vi "Untitled 2.vi"() -> ()   [LabVIEW 2016]
uses:
  <userlib>/LevyLab/XY Utilities/Typedefs/Interpolation Configuration--cluster.ctl
  <userlib>/LevyLab/Graph Utilities/graph_utilities.lvclass
  <userlib>/LevyLab/Graph Utilities/graph_utilities.lvclass/graph_utilities.ctl
  <userlib>/LevyLab/Graph Utilities/XY Graph/Set XY Graph Value (array).vi
  <userlib>/LevyLab/XY Utilities/subVIs/Add float (multiple).vi
  <userlib>/LevyLab/XY Utilities/subVIs/Subtract float (multiple).vi
  <userlib>/LevyLab/XY Utilities/subVIs/Multiply float (multiple).vi
  <userlib>/LevyLab/XY Utilities/subVIs/Square (multiple).vi
  <userlib>/LevyLab/XY Utilities/subVIs/Divide float (multiple).vi
  <userlib>/LevyLab/XY Utilities/subVIs/Sort (multiple).vi
  <userlib>/LevyLab/XY Utilities/subVIs/Swap X and Y (multiple).vi
  <userlib>/LevyLab/XY Utilities/subVIs/Reverse (multiple).vi
  <userlib>/LevyLab/XY Utilities/subVIs/Subset (multiple).vi
  <userlib>/LevyLab/XY Utilities/subVIs/Derivative (multiple).vi
  <userlib>/LevyLab/XY Utilities/subVIs/Interpolate (multiple).vi
  <userlib>/LevyLab/XY Utilities/subVIs/FFT (multiple).vi
  <userlib>/LevyLab/XY Utilities/subVIs/PS (multiple).vi
  <userlib>/LevyLab/XY Utilities/subVIs/Resample (multiple).vi
  <userlib>/LevyLab/XY Utilities/subVIs/Symmetrize (multiple).vi
  <userlib>/LevyLab/XY Utilities/xy_utilities.lvlib
  <userlib>/LevyLab/LV to ITX/Data.TDMS/Data.TDMS.lvclass
  <userlib>/LevyLab/XY Utilities/subVIs/Add XY (multiple).vi
panel:
  in  "Tab Control":enum32{"Page 1", "Page 2"}(tab)
  in  "STOP":bool
  in  "CLEAR":bool
  out "Current State":string="XY: Load\nGraph: Initialize Graphs\nUI: Display Data"
  in  "Method":enum16{"Slider (%)", "X[] min and max"}(ring)
  in  "Subset Slider":cluster{dbl, dbl}(slide)={0.75, 0.25} caption="Horizontal Slider" scale=0.0..1.0
  in  "Interval":dbl=2.0
  in  "Type":enum16{"dy/dx vs x", "dx/dy vs y"}(ring)
  in  "PROCESS":bool
  in  "Process Queue":string
  in  "Available States":i32(listbox)=-1 caption="States to Process"
  in  "x":dbl format="%#_6p"
  in  "y":dbl format="%#_6p"
  out "Processed States":string="XY: Load\nGraph: Initialize Graphs\nUI: Display Data"
  in  "Interval Units":enum16{"Points", "Data"}(ring)
  in  "Configure":T1={"X Low"=0.05, "X High"=0.5, "X Step"=0.01, "Fake Point"=0.05} {"Fake Point" format="%#_6p"; "X Step" format="%#_6p"; "X High" format="%#_6p"; "X Low" format="%#_6p"}
  in  "File or Folder Path":path=path "C:/"
  in  "Channels":cluster{"X":string, "Y":string, "N":string}
  in  "Numeric":i32
  out "counter":i32
  in  "Graphs Tab Control":enum32{"Data", "Intensity/Linecuts"}(tab)
  out "XY Graph: Antisymmetric":cluster{"X-array":dbl[], dbl[]}[](graph)
  out "XY Graph: Symmetric":cluster{"X-array":dbl[], dbl[]}[](graph)
  out "XY Graph: Processed":cluster{"Intensity Data":dbl[], "Array":dbl[]}[](graph)
  out "XY Graph: Unprocessed":cluster{"Intensity Data":dbl[], "Array":dbl[]}[](graph)
  out "Data Intensity":dbl[][](graph)
  out "Diff Intensity":dbl[][](graph)
  out "Diff Vertical":cluster{"Array":dbl[], "A x Vector":dbl[]}[](graph)
  out "Diff Horizontal":cluster{"Array":dbl[], "A x Vector":dbl[]}[](graph)
  in  "width (vertical)":dbl=0.2 caption="width"
  in  "width (horizontal)":dbl=0.2 caption="width"
  in  "width (vertical) 2":dbl=0.2 caption="width"
  in  "width (horizontal) 2":dbl=0.2 caption="width"
  out "Data Vertical":cluster{"Array":dbl[], "A x Vector":dbl[]}[](graph)
  out "Data Horizontal":cluster{"Intensity Data":dbl[], "Array":dbl[]}[](graph)
  # "State Scripting"
  # "Process Arguments"
  # "Arithmetic"
  # "Derivative"
  # "Interpolate"
  # "Subset"
  # "\"Process Queue\" is a list of states that will execute when you press the \"PROCESS\" button. (File: Load and Graph: Update Graph are added automatically to the beginning and end of the queue.)\n\nTo add states you can either:\n- Type directly into the Process Queue box.\nor:\n- Select a state in the \"Available States\" box that you want to add to the queue. ctl-v in the \"Process Queue\" control to add to the queue."
  # "XY Graphs"
  # "Symmeterized Graphs"
  # "Data processing (1)"
  # "Data Processing (2)"
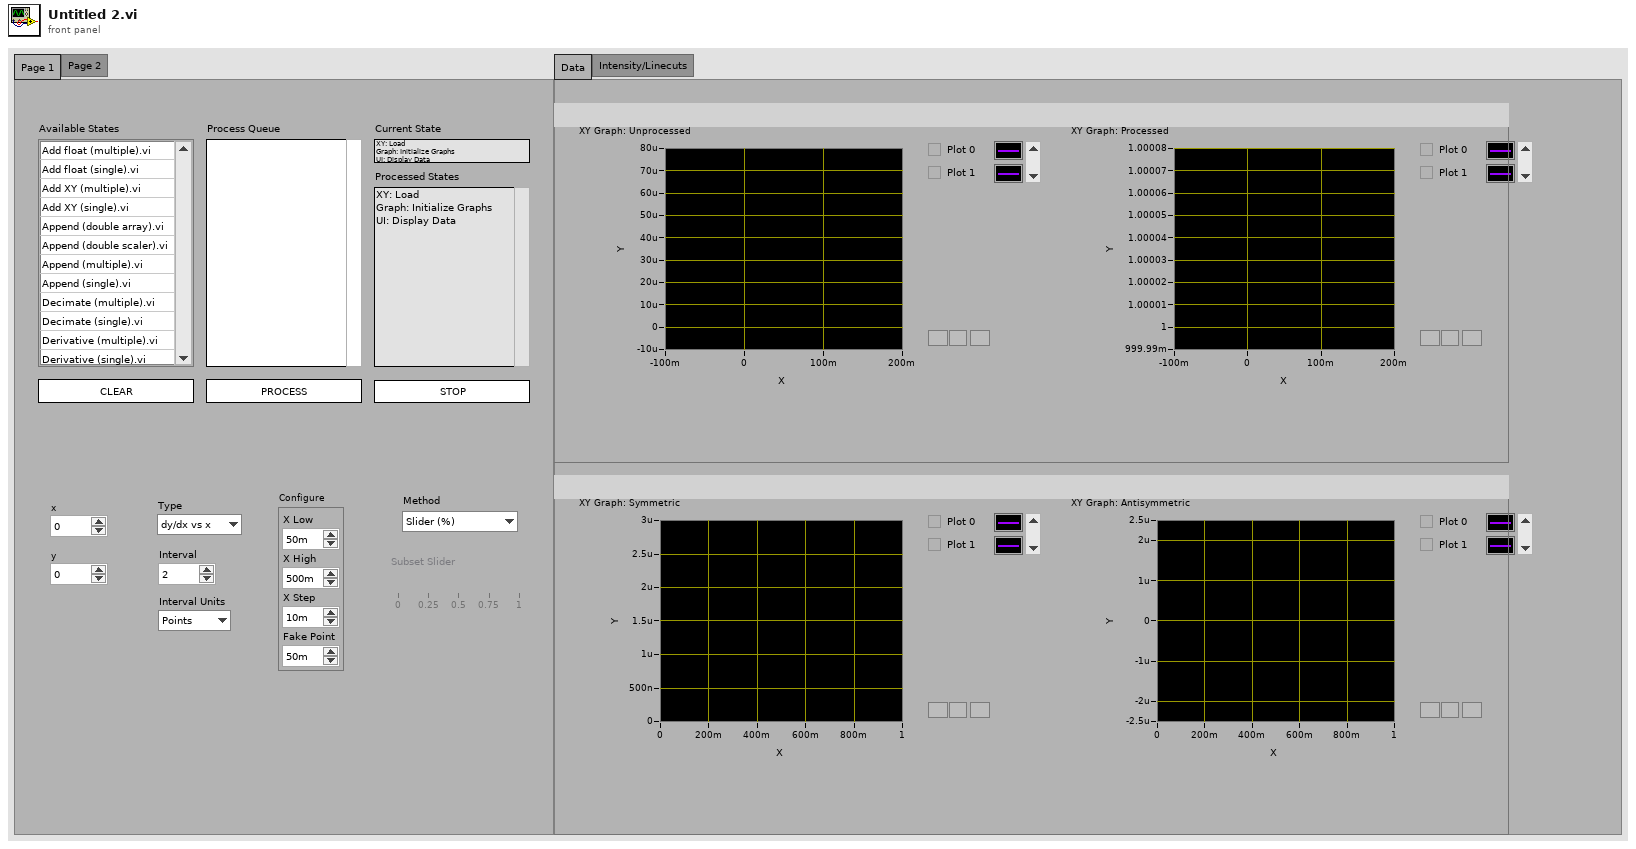
[diagram p1: front panel]
types:
  T1 = typedef "xy_utilities.lvlib/Interpolation Configuration--cluster.ctl" = cluster{"X Low":dbl, "X High":dbl, "X Step":dbl, "Fake Point":dbl}
  T2 = enum32{"Invalid", "Standard", "Closed", "Hidden", "Minimized", "Maximized"}
  T3 = enum32{"invalid app kind", "Development System", "Run Time System", "Student Edition", "Embedded LabVIEW", "Evaluation", "Custom"}
  T4 = cluster{"Shift":bool, "Ctrl":bool, "Alt":bool, "Cmd":bool, "Opt":bool}
  T5 = cluster{"Core":cluster{"Current VI Reference":refnum<vi>, "Close Panel on Exit?":bool}, "Graph":cluster{"Data: Unprocessed":refnum<class "graph_utilities.lvclass">, "Data: Processed":refnum<class "graph_utilities.lvclass">, "Data: Intensity/Vertical":refnum<class "graph_utilities.lvclass">, "Data: Intensity/Horizontal":refnum<class "graph_utilities.lvclass">, "Differential: Intensity/Vertical":refnum<class "graph_utilities.lvclass">, "Differential: Intensity/Horizontal":refnum<class "graph_utilities.lvclass">}, "XY Data (unprocessed)":cluster{"Intensity Data":dbl[], "Array":dbl[]}[], "XY Data (processed 1)":cluster{"Intensity Data":dbl[], "Array":dbl[]}[], "XY Data (processed 2)":cluster{"Intensity Data":dbl[], "Array":dbl[]}[], "Parameter":dbl[]}
  T6 = cluster{"Data: Unprocessed":refnum<class "graph_utilities.lvclass">, "Data: Processed":refnum<class "graph_utilities.lvclass">, "Data: Intensity/Vertical":refnum<class "graph_utilities.lvclass">, "Data: Intensity/Horizontal":refnum<class "graph_utilities.lvclass">, "Differential: Intensity/Vertical":refnum<class "graph_utilities.lvclass">, "Differential: Intensity/Horizontal":refnum<class "graph_utilities.lvclass">}
  T7 = cluster{"Current VI Reference":refnum<vi>, "Close Panel on Exit?":bool}
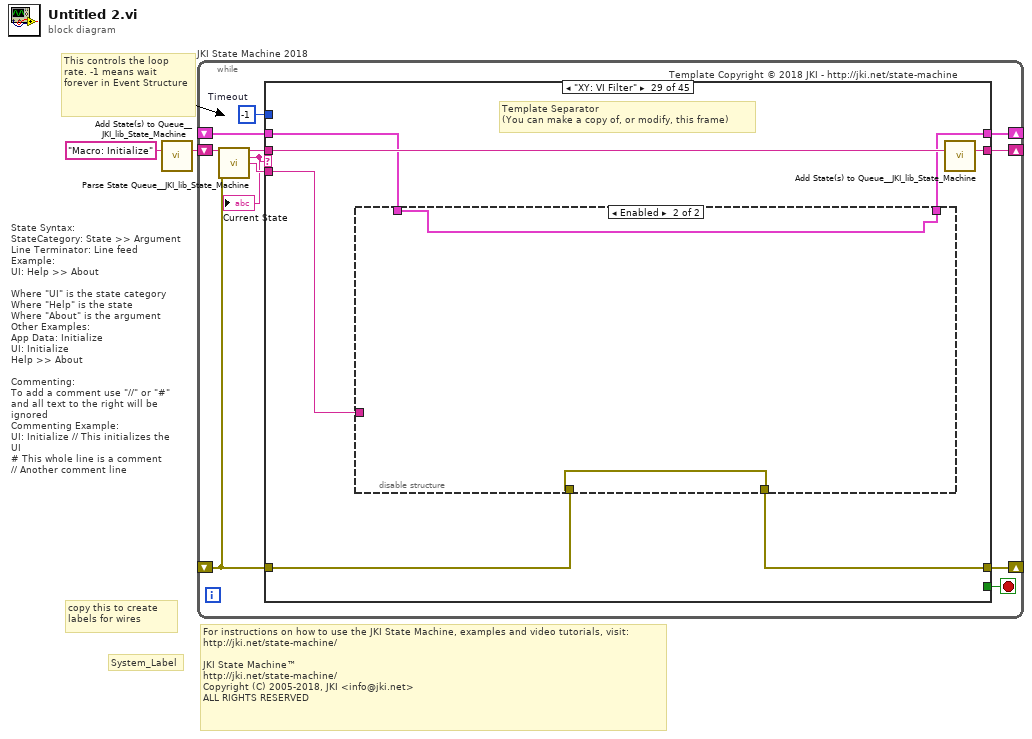
[diagram p0: block diagram]
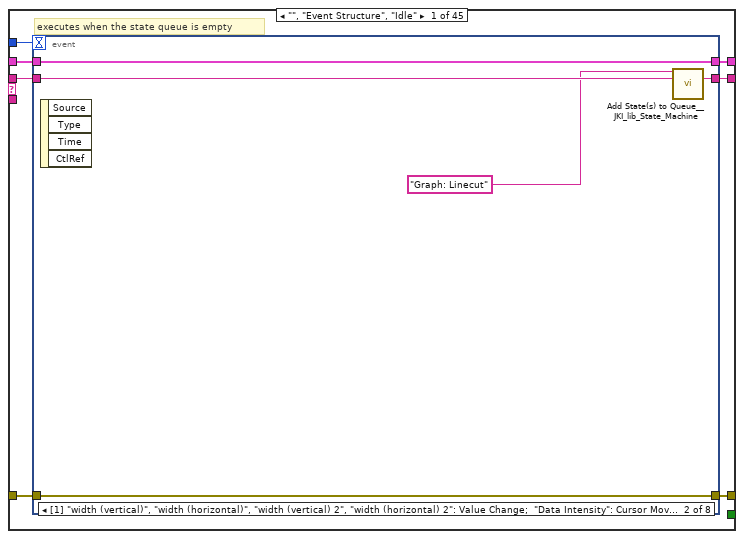
[diagram p2: hidden frame]
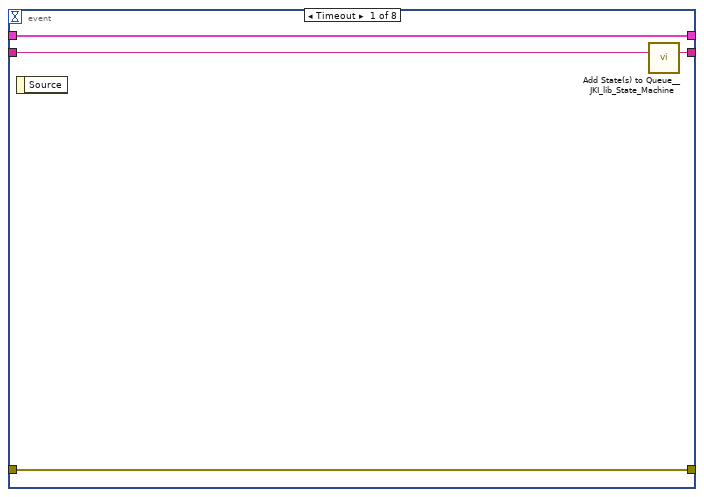
[diagram p3: hidden frame]
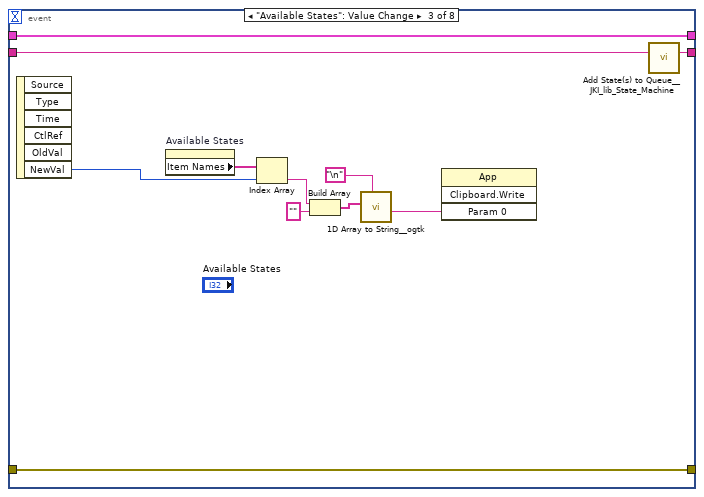
[diagram p4: hidden frame]
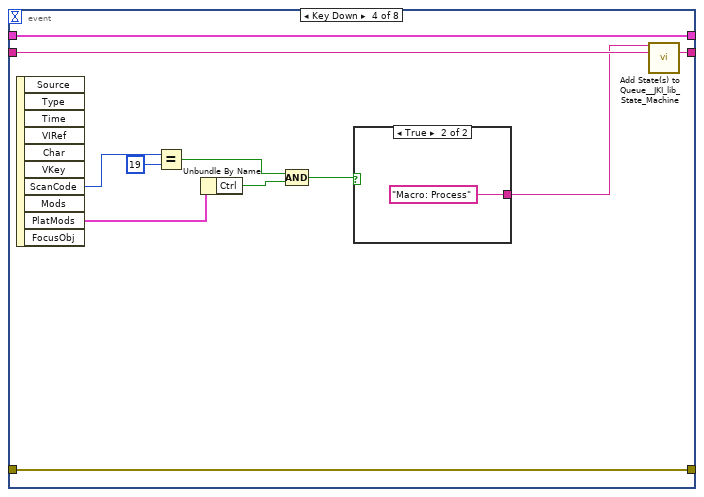
[diagram p5: hidden frame]
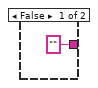
[diagram p6: hidden frame]
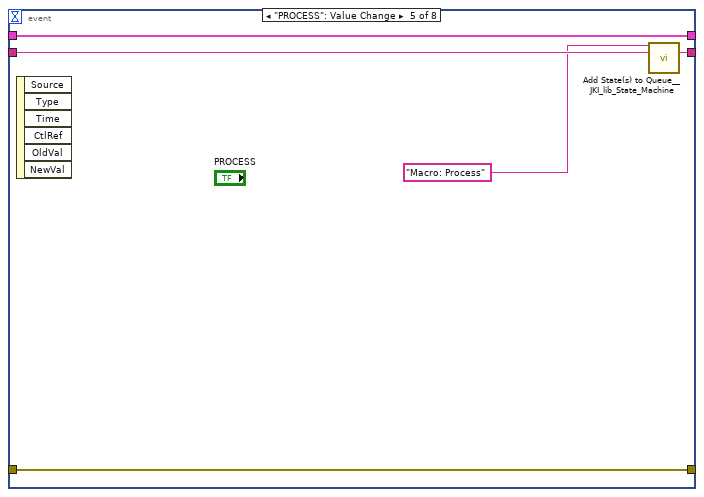
[diagram p7: hidden frame]
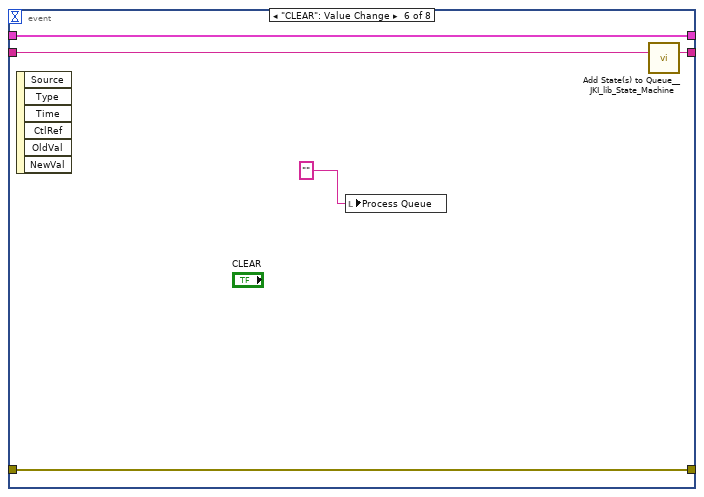
[diagram p8: hidden frame]
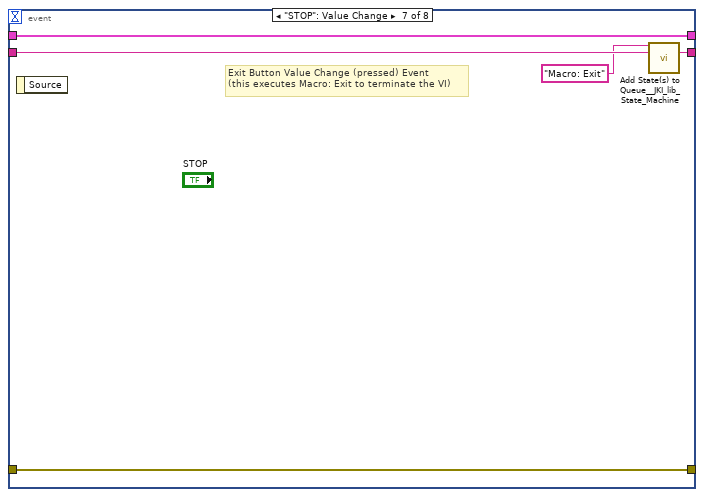
[diagram p9: hidden frame]
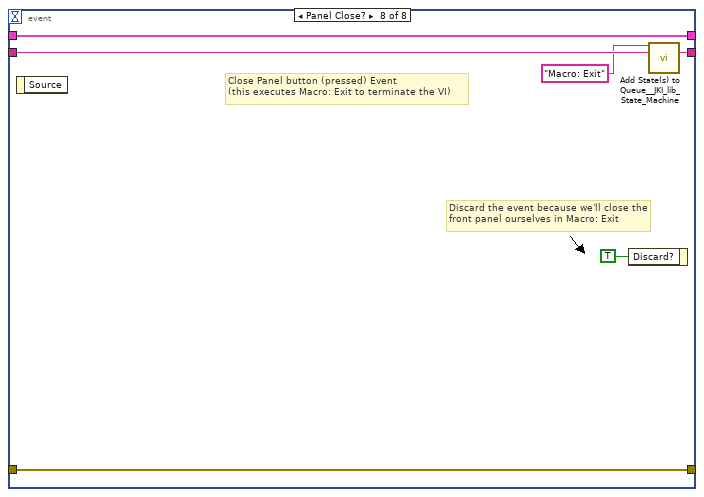
[diagram p10: hidden frame]
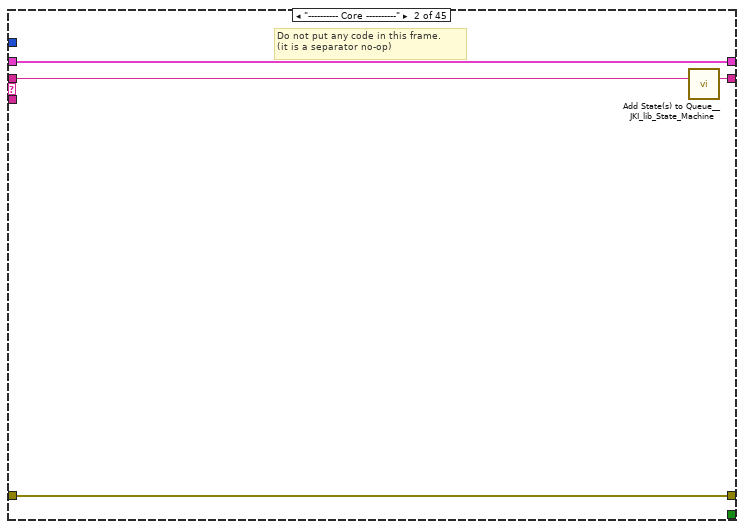
[diagram p11: hidden frame]
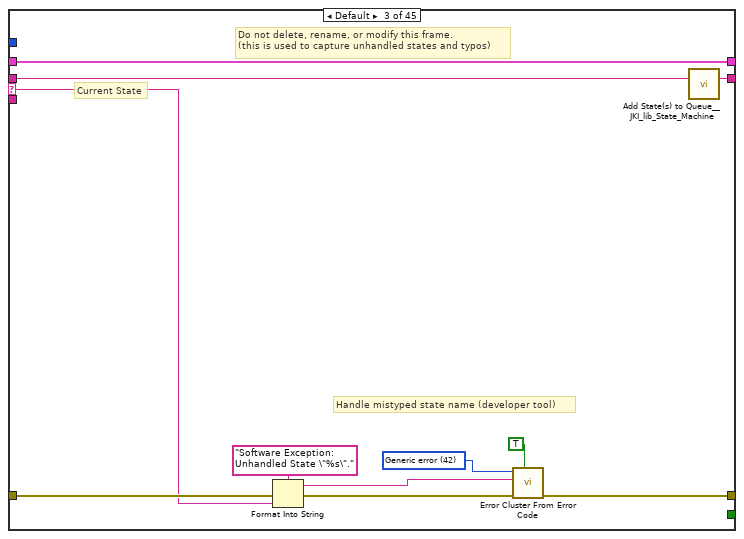
[diagram p12: hidden frame]
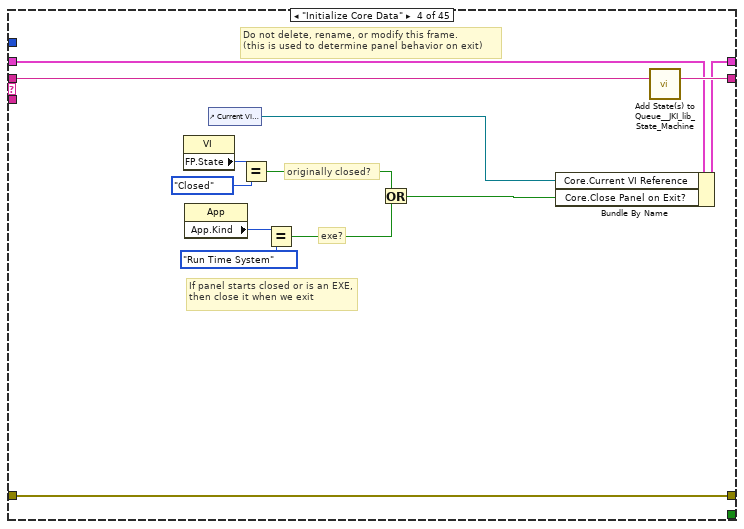
[diagram p13: hidden frame]
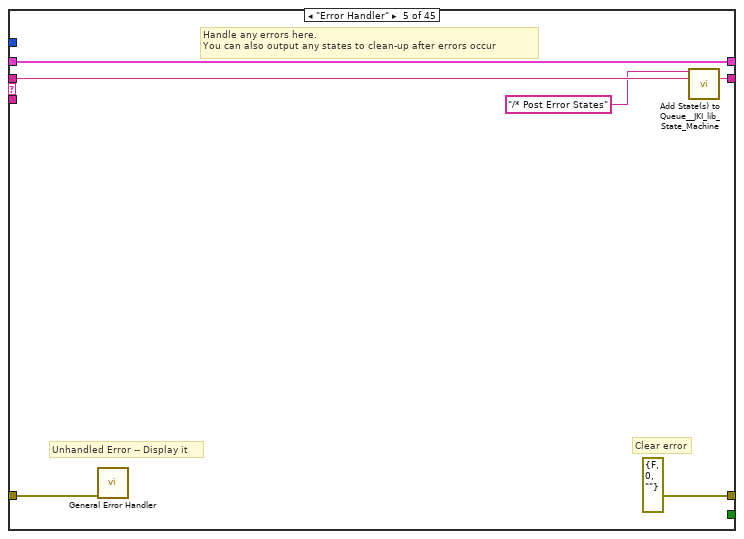
[diagram p14: hidden frame]
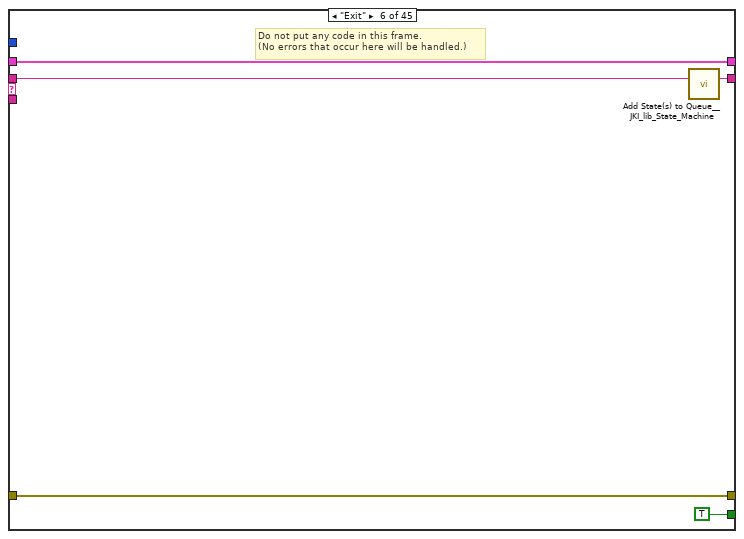
[diagram p15: hidden frame]
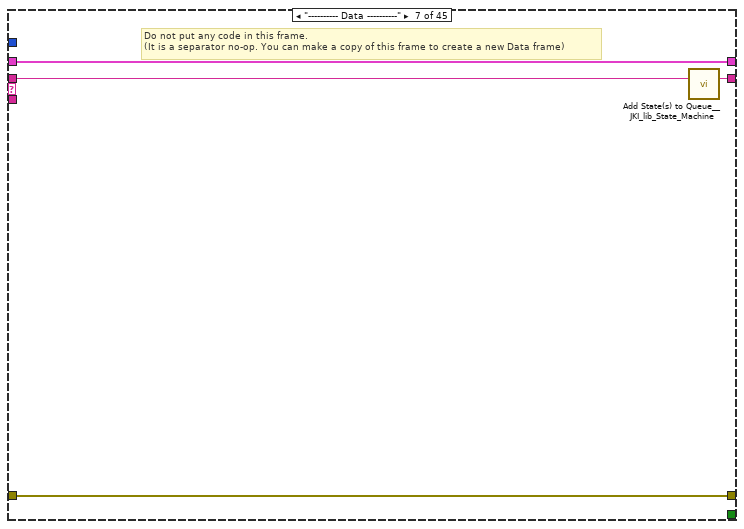
[diagram p16: hidden frame]
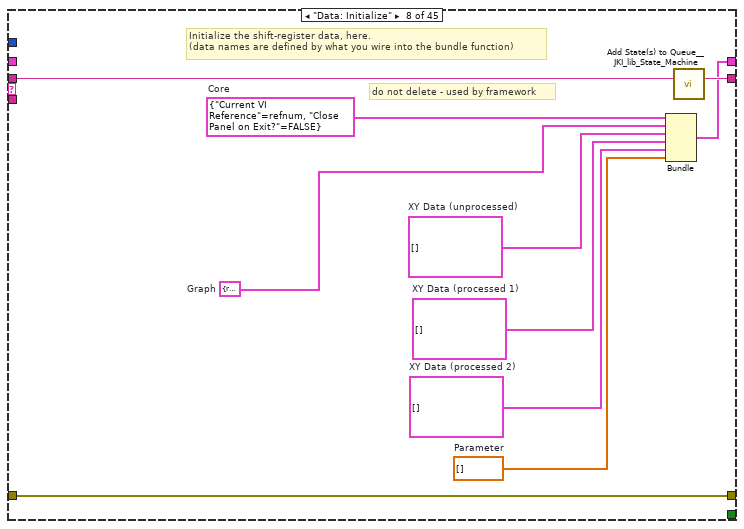
[diagram p17: hidden frame]
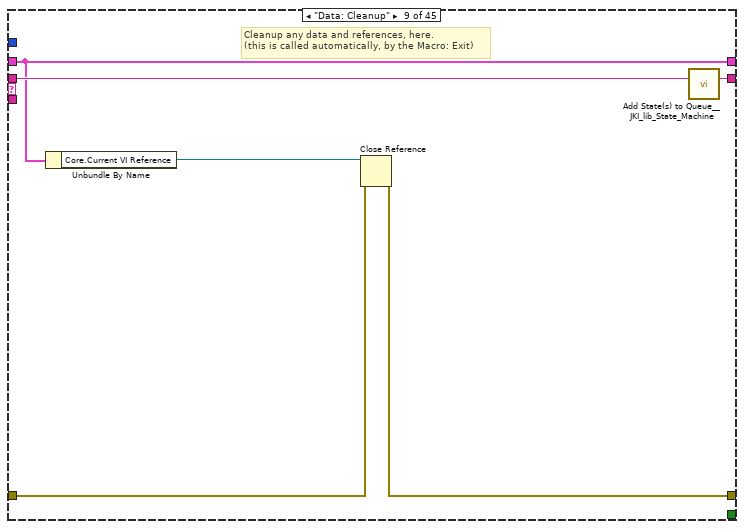
[diagram p18: hidden frame]
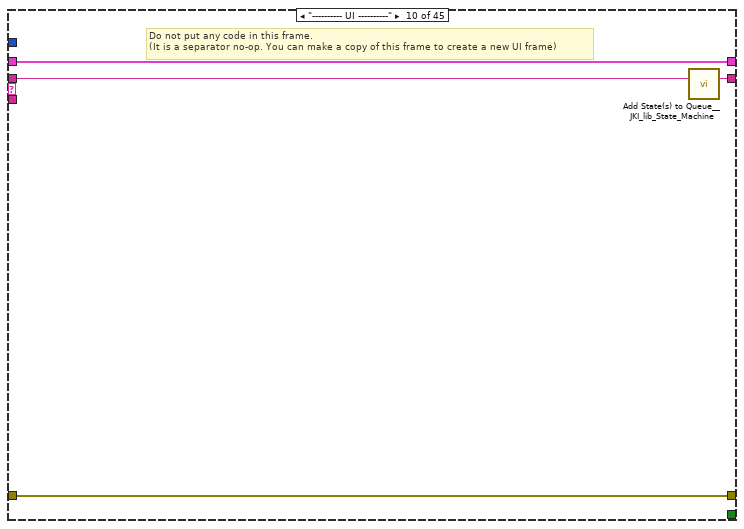
[diagram p19: hidden frame]
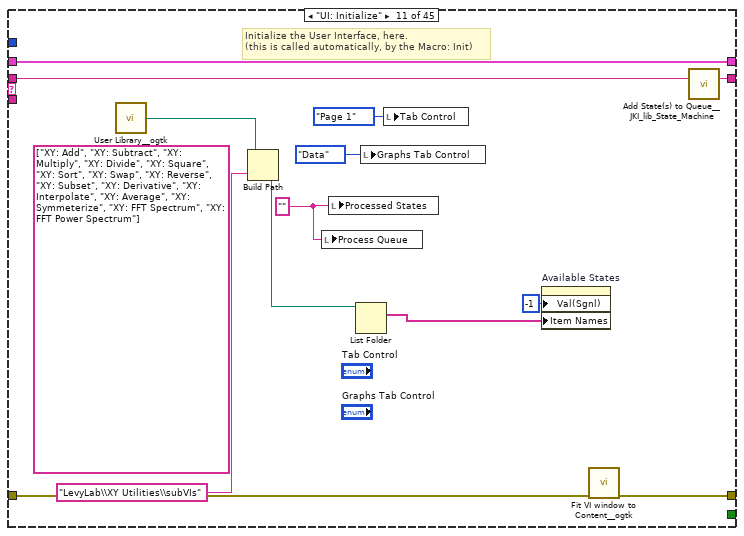
[diagram p20: hidden frame]
diagram:
  # "For instructions on how to use the JKI State Machine, examples and video tutorials, visit:\nhttp://jki.net/state-machine/\n\nJKI State Machine™\nhttp://jki.net/state-machine/\nCopyright (C) 2005-2018, JKI <info@jki.net>\nALL RIGHTS RESERVED"
  # "State Syntax:\nStateCategory: State >> Argument\nLine Terminator: Line feed\nExample:\nUI: Help >> About\n\nWhere \"UI\" is the state category\nWhere \"Help\" is the state\nWhere \"About\" is the argument\nOther Examples:\nApp Data: Initialize\nUI: Initialize\nHelp >> About\n\nCommenting:\nTo add a comment use \"//\" or \"#\" and all text to the right will be ignored\nCommenting Example:\nUI: Initialize // This initializes the UI\n# This whole line is a comment\n// Another comment line"
  # "copy this to create labels for wires"
  # "This controls the loop rate. -1 means wait forever in Event Structure"
  # "System_Label"
  n1 = call <vilib>:"Add State(s) to Queue__JKI_lib_State_Machine.vi"("State(s) in (\"\")"="Macro: Initialize") -> ("States Out"=w1:string)  [unwired: 14 in]
  n2 = while "JKI State Machine 2018" {
    shift-right: [w7] -> _
    shift-left: _ -> [w6]
    shift-right: [w10] -> _
    shift-left: _ -> [w4]
    shift-right: [w9] -> _
    shift-left: w1 -> [w11]
    stop <- w8 stop-if-true
    w5 = -1  # Timeout
    # "Template Copyright © 2018 JKI - http://jki.net/state-machine"
    n3 = call <vilib>:"Parse State Queue__JKI_lib_State_Machine.vi"("State Queue"=w11, "Error In (no error)"=w4) -> ("Remaining States"=w13:string, "Current State"=w3:string, "Arguments"=w12:string)  [unwired: 11 in]
    "Current State" <- w3
    n4 = case shown="\"XY: VI Filter\"" w3 {
      selector: w3 -> [_ _ w79 _ _ _ _ _ _ _ _ _ _ _ _ _ _ _ _ _ _ _ _ _ _ _ _ _ _ _ _ _ _ _ _ _ _ _ _ _ _ _ _ _ _]
      tunnel: w13 -> [w20 w78 w83 w102 w108 w113 w117 w127 w133 w137 w150 w156 w167 w236 w241 w251 w261 w265 w269 w286 w310 w320 w330 w354 w370 w374 w387 w410 w417 w446 w456 w466 w474 w484 w492 w500 w508 w518 w529 w538 w546 w554 w562 w570 w580]
      tunnel: w12 -> [_ _ _ _ _ _ _ _ _ _ _ w151 w161 _ _ _ _ _ _ _ _ _ _ _ _ _ _ _ w413 _ _ _ _ _ _ _ _ _ _ _ _ _ _ _ _]
      tunnel: w6 -> [w18 w75 w81 w95 w105 w111 w114 _ w128 w134 w148 w154 w163 w233 w238 w248 w258 w262 w266 w284 w308 w315 w328 w351 w368 w371 w384 w407 w415 w443 w453 w463 w471 w481 w489 w497 w505 w515 w526 w535 w543 w551 w559 w567 w577]
      tunnel: [w17 w76 w85 w99 errorcluster {"status"=FALSE, "code"=0, "source"=""} ("error out") w110 w115 w124 w129 w135 w142 w152 w164 w234 w239 w249 w259 w263 w267 w282 w293 w311 w321 w352 w359 w372 w383 w403 w411 w439 w449 w459 w467 w477 w485 w493 w501 w511 w523 w531 w539 w548 w555 w563 w573] -> w10
      tunnel: w4 -> [w16 w76 w84 w99 w104 w110 w115 w124 w130 w135 w143 w153 w165 w234 w239 w249 w259 w263 w267 w273 w287 w314 w325 w352 w361 w372 w383 w404 w412 w440 w450 w460 w468 w478 w486 w494 w502 w512 w524 w532 w540 w549 w556 w564 w574]
      tunnel: [w19 w77 w82 w101 w107 w112 w116 w126 w132 w136 w149 w155 w166 w235 w240 w250 w260 w264 w268 w285 w309 w319 w329 w353 w369 w373 w386 w409 w416 w445 w455 w465 w473 w483 w491 w499 w507 w517 w528 w537 w545 w553 w561 w569 w579] -> w9
      tunnel: [_ _ _ _ _ TRUE _ _ _ _ _ _ _ _ _ _ _ _ _ _ _ _ _ _ _ _ _ _ _ _ _ _ _ _ _ _ _ _ _ _ _ _ _ _ _] -> w8
      tunnel: [w15 w75 w81 w100 w105 w111 w114 w125 w128 w134 w148 w154 w163 w233 w238 w248 w258 w262 w266 w283 w307 w315 w328 w351 w368 w371 w385 w406 w414 w442 w452 w462 w470 w480 w488 w496 w504 w514 w525 w534 w542 w550 w558 w566 w576] -> w7
      tunnel: w5 -> [w14 _ _ _ _ _ _ _ _ _ _ _ _ _ _ _ _ _ _ _ _ _ _ _ _ _ _ _ _ _ _ _ _ _ _ _ _ _ _ _ _ _ _ _ _]
      frame "", "Event Structure", "Idle" {
        # "executes when the state queue is empty"
        n5 = event shown="[1] \"width (vertical)\", \"width (horizontal)\", \"width (vertical) 2\", \"width (horizontal) 2\": Value Change;  \"Data Intensity\": Cursor Move" {
          selector: _ -> [_ _ _ _ _ _ _ _]
          dyn-events: _ -> [_ _ _ _ _ _ _ _]
          timeout: w14 -> [_ _ _ _ _ _ _ _]
          tunnel: w20 -> [w24 w29 w40 w51 w58 w63 w68 w74]
          tunnel: [w23 w28 w39 w50 w57 w62 w67 w73] -> w19
          tunnel: w18 -> [w21 w26 w37 w48 w55 w60 w65 w71]
          tunnel: [w22 w27 w38 w49 w56 w61 w66 w72] -> w17
          tunnel: w16 -> [w22 w27 w38 w49 w56 w61 w66 w72]
          tunnel: [w21 w26 w37 w48 w55 w60 w65 w71] -> w15
          event Timeout {
            n6 = event-data() -> ()  [unwired: 1 in, 1 out]
            n7 = call <vilib>:"Add State(s) to Queue__JKI_lib_State_Machine.vi"("State(s) in (\"\")"=w24) -> ("States Out"=w23:string)  [unwired: 14 in]
          }
          event "width (vertical)", "width (horizontal)", "width (vertical) 2", "width (horizontal) 2": Value Change; "Data Intensity": Cursor Move {
            n8 = event-data() -> ()  [unwired: 1 in, 4 out]
            n9 = call <vilib>:"Add State(s) to Queue__JKI_lib_State_Machine.vi"("State(s) in Front (\"\")"="Graph: Linecut" ("State(s) in Front (\"\")"), "State(s) in (\"\")"=w29) -> ("States Out"=w28:string)  [unwired: 13 in]
          }
          event "Available States": Value Change {
            n10 = event-data() -> ("NewVal"=w31:i32)  [unwired: 1 in, 5 out]
            n11 = property on="Available States" class="LstBox (strict)"() -> ("Item Names"=w32:string[])  [unwired: 2 in, 2 out]
            n12 = Index Array(array=w32, index=w31) -> (element=w36:string)
            n13 = Build Array(w36, "" ("element")) -> (w33:string[])
            n14 = call <userlib>:"1D Array to String__ogtk.vi"("delimiter (Tab)"="\n", "Array of Strings"=w33) -> ("delimited string"=w34:string)  [unwired: 9 in]
            n15 = invoke class="App" method="Clipboard.Write"("Param 0"=w34) -> ()  [unwired: 3 in, 4 out]
            n16 = call <vilib>:"Add State(s) to Queue__JKI_lib_State_Machine.vi"("State(s) in (\"\")"=w40) -> ("States Out"=w39:string)  [unwired: 14 in]
          }
          event Key Down {
            n17 = event-data() -> ("ScanCode"=w41:i16, "PlatMods"=w42:T4)  [unwired: 1 in, 8 out]
            n18 = Equal?(x=w41, y=i16 19) -> (x = y?=w44:bool)
            n19 = Unbundle By Name(w42) -> ("Ctrl"=w45:bool)
            n20 = Compound Arithmetic op=AND(w44, w45) -> (w43:bool)
            n21 = case shown="True" w43 {
              tunnel: ["" ("State(s) in Front (\"\")") "Macro: Process" ("State(s) in Front (\"\")")] -> w46
              frame False {
              }
              frame True {
              }
            }
            n22 = call <vilib>:"Add State(s) to Queue__JKI_lib_State_Machine.vi"("State(s) in Front (\"\")"=w46, "State(s) in (\"\")"=w51) -> ("States Out"=w50:string)  [unwired: 13 in]
          }
          event "PROCESS": Value Change {
            n23 = event-data() -> ()  [unwired: 1 in, 6 out]
            n24 = call <vilib>:"Add State(s) to Queue__JKI_lib_State_Machine.vi"("State(s) in Front (\"\")"="Macro: Process" ("State(s) in Front (\"\")"), "State(s) in (\"\")"=w58) -> ("States Out"=w57:string)  [unwired: 13 in]
          }
          event "CLEAR": Value Change {
            n25 = event-data() -> ()  [unwired: 1 in, 6 out]
            n26 = local write "Process Queue"("" ("Process States")) -> ()
            n27 = call <vilib>:"Add State(s) to Queue__JKI_lib_State_Machine.vi"("State(s) in (\"\")"=w63) -> ("States Out"=w62:string)  [unwired: 14 in]
          }
          event "STOP": Value Change {
            # "Exit Button Value Change (pressed) Event\n(this executes Macro: Exit to terminate the VI)"
            n28 = event-data() -> ()  [unwired: 1 in, 1 out]
            n29 = call <vilib>:"Add State(s) to Queue__JKI_lib_State_Machine.vi"("State(s) in Front (\"\")"="Macro: Exit", "State(s) in (\"\")"=w68) -> ("States Out"=w67:string)  [unwired: 13 in]
          }
          event Panel Close? {
            # "Discard the event because we'll close the front panel ourselves in Macro: Exit"
            # "Close Panel button (pressed) Event\n(this executes Macro: Exit to terminate the VI)"
            n30 = event-data() -> ()  [unwired: 1 in, 1 out]
            n31 = event-data("Discard?"=TRUE) -> ()  [unwired: 1 in, 1 out]
            n32 = call <vilib>:"Add State(s) to Queue__JKI_lib_State_Machine.vi"("State(s) in Front (\"\")"="Macro: Exit", "State(s) in (\"\")"=w74) -> ("States Out"=w73:string)  [unwired: 13 in]
          }
        }
      }
      frame "---------- Core ----------" {
        # "Do not put any code in this frame.\n(it is a separator no-op)"
        n33 = call <vilib>:"Add State(s) to Queue__JKI_lib_State_Machine.vi"("State(s) in (\"\")"=w78) -> ("States Out"=w77:string)  [unwired: 14 in]
      }
      frame Default {
        w88 = 42 items=["No error", "Argument error", "Memory is full", "Out of zone", "End of file", "File already open", "Generic file I/O error", "File not found", "File permission error", "Disk is full", "Duplicate path", "Too many files open", "System feature not enabled", "Resource file not found", "Cannot add resource", "Resource not found", "Image not found", "Image memory error", "Pen does not exist", "Config type invalid", "Config token not found", "Config parse error", "Config memory error", "Bad external code format", "Bad external code offset", "External code not present", "Null window", "Destroy window error", "Null menu", "Print aborted", "Bad print record", "Print driver error", "Windows error during printing", "Memory error during printing", "Print dialog error", "Generic print error", "Invalid device refnum", "Device not found", "Device parameter error", "Device unit error", "Cannot open device", "Device call aborted", "Generic error", "Cancelled by user", "Object ID too low", "Object ID too high", "Object not in heap", "Unknown heap", "Unknown object (invalid DefProc)", "Unknown object (DefProc not in table)", "Message out of range", "Invalid (null) method", "Unknown message", "Manager call not supported", "Bad address", "Network operation in progress", "Network operation timed out", "Connection is busy", "Network attribute not supported", "Network error", "Address in use", "System out of memory", "Connection aborted", "Connection refused", "Not connected", "Already connected", "Connection closed", "Initialization error (interapplication manager)", "Bad occurrence", "Wait on unbound occurrence handler", "Occurrence queue overflow", "Datalog type conflict", "Unused", "Unrecognized type (interapplication manager)", "Memory corrupt", "Failed to make temporary DLL", "Old CIN version", "Drag socket not found", "Failed to load drop-object", "Failed to register OLE object", "Failed to release OLE object", "Format specifier type mismatch", "Unknown format specifier", "Too few format specifiers", "Too many format specifiers", "Scan failed", "Newer CIN version", "Error converting to variant", "Runtime menu error", "Password tampered", "Variant attribute not found", "Incompatible variant data type", "Event data is not available", "Event Store is not present", "Occurrence is not found", "Event Queue is not created", "Event info is not available", "Refnum passed is NULL", "Error retrieving Class GUID", "Error retrieving CoClass GUID", "Error retrieving TypeLib GUID.", "Bad built application magic bytes.", "Specific driver is different from the specific driver associated with the Logical Name.", "There is no session opened to the class driver.", "Max Error", "MAX - Error with config objects", "MAX - Error loading configuration", "MAX - Group not supported"]
        # "Current State"
        # "Do not delete, rename, or modify this frame.\n(this is used to capture unhandled states and typos)"
        # "Handle mistyped state name (developer tool)"
        n34 = Format Into String(format string="Software Exception: Unhandled State \"%s\"." ("message"), error in=w84, w79) -> (resulting string=w87:string, error out=w86:errorcluster)  [unwired: 1 in]
        n35 = call <vilib>:"Error Cluster From Error Code.vi"("show call chain? (False)"=TRUE, "error in (no error)"=w86, "error message (\"\")"=w87, "error code (0)"=w88) -> ("error out"=w85:errorcluster)  [unwired: 5 in]
        n36 = call <vilib>:"Add State(s) to Queue__JKI_lib_State_Machine.vi"("State(s) in (\"\")"=w83) -> ("States Out"=w82:string)  [unwired: 14 in]
      }
      frame "Initialize Core Data" {
        # "Do not delete, rename, or modify this frame.\n(this is used to determine panel behavior on exit)"
        # "originally closed?"
        # "exe?"
        # "If panel starts closed or is an EXE, then close it when we exit"
        n37 = property class="VI"() -> ("FP.State"=w92:T2)  [unwired: 2 in, 2 out]
        n38 = property class="App"() -> ("App.Kind"=w98:T3)  [unwired: 2 in, 2 out]
        n39 = control-ref of="Current VI Reference"() -> (w93:refnum<vi>)
        n40 = Equal?(x=w92, y=T2."Closed" ("Front Panel Window:State")) -> (x = y?=w90:bool)
        n41 = Equal?(x=w98, y=T3."Run Time System" ("Application:Kind")) -> (x = y?=w96:bool)
        n42 = Or(x=w90, y=w96) -> (x .or. y?=w94:bool)
        n43 = Bundle By Name(cluster=w95, "Core.Current VI Reference"=w93, "Core.Close Panel on Exit?"=w94) -> (w100:T5)
        n44 = call <vilib>:"Add State(s) to Queue__JKI_lib_State_Machine.vi"("State(s) in (\"\")"=w102) -> ("States Out"=w101:string)  [unwired: 14 in]
      }
      frame "Error Handler" {
        # "Unhandled Error -- Display it"
        # "Handle any errors here.\nYou can also output any states to clean-up after errors occur"
        # "Clear error"
        n45 = call <vilib>:"General Error Handler.vi"("error in (no error)"=w104) -> ()  [unwired: 10 in, 5 out]
        n46 = call <vilib>:"Add State(s) to Queue__JKI_lib_State_Machine.vi"("State(s) in Front (\"\")"="/* Post Error States", "State(s) in (\"\")"=w108) -> ("States Out"=w107:string)  [unwired: 13 in]
      }
      frame "Exit" {
        # "Do not put any code in this frame.\n(No errors that occur here will be handled.)"
        n47 = call <vilib>:"Add State(s) to Queue__JKI_lib_State_Machine.vi"("State(s) in (\"\")"=w113) -> ("States Out"=w112:string)  [unwired: 14 in]
      }
      frame "---------- Data ----------" {
        # "Do not put any code in this frame.\n(It is a separator no-op. You can make a copy of this frame to create a new Data frame)"
        n48 = call <vilib>:"Add State(s) to Queue__JKI_lib_State_Machine.vi"("State(s) in (\"\")"=w117) -> ("States Out"=w116:string)  [unwired: 14 in]
      }
      frame "Data: Initialize" {
        w118 = T6 {"Data: Unprocessed"=refnum, "Data: Processed"=refnum, "Data: Intensity/Vertical"=refnum, "Data: Intensity/Horizontal"=refnum, "Differential: Intensity/Vertical"=refnum, "Differential: Intensity/Horizontal"=refnum}  # Graph
        w119 = cluster{"Intensity Data":dbl[], "Array":dbl[]}[] []  # XY Data (processed 2)
        w120 = dbl[] []  # Parameter
        w121 = cluster{"Intensity Data":dbl[], "Array":dbl[]}[] []  # XY Data (processed 1)
        w122 = cluster{"Intensity Data":dbl[], "Array":dbl[]}[] []  # XY Data (unprocessed)
        w123 = T7 {"Current VI Reference"=refnum, "Close Panel on Exit?"=FALSE}  # Core
        # "do not delete - used by framework"
        # "Initialize the shift-register data, here.\n(data names are defined by what you wire into the bundle function)"
        n49 = Bundle("Core"=w123, "Graph"=w118, "XY Data (unprocessed)"=w122, "XY Data (processed 1)"=w121, "XY Data (processed 2)"=w119, "Parameter"=w120) -> (w125:T5)  [unwired: 1 in]
        n50 = call <vilib>:"Add State(s) to Queue__JKI_lib_State_Machine.vi"("State(s) in (\"\")"=w127) -> ("States Out"=w126:string)  [unwired: 14 in]
      }
      frame "Data: Cleanup" {
        # "Cleanup any data and references, here.\n(this is called automatically, by the Macro: Exit)"
        n51 = Unbundle By Name(w128) -> ("Core.Current VI Reference"=w131:refnum<vi>)
        n52 = Close Reference(reference=w131, error in (no error)=w130) -> (error out=w129:errorcluster)
        n53 = call <vilib>:"Add State(s) to Queue__JKI_lib_State_Machine.vi"("State(s) in (\"\")"=w133) -> ("States Out"=w132:string)  [unwired: 14 in]
      }
      frame "---------- UI ----------" {
        # "Do not put any code in this frame.\n(It is a separator no-op. You can make a copy of this frame to create a new UI frame)"
        n54 = call <vilib>:"Add State(s) to Queue__JKI_lib_State_Machine.vi"("State(s) in (\"\")"=w137) -> ("States Out"=w136:string)  [unwired: 14 in]
      }
      frame "UI: Initialize" {
        (unwired) string[] ["XY: Add", "XY: Subtract", "XY: Multiply", "XY: Divide", "XY: Square", "XY: Sort", "XY: Swap", "XY: Reverse", "XY: Subset", "XY: Derivative", "XY: Interpolate", "XY: Average", "XY: Symmeterize", "XY: FFT Spectrum", "XY: FFT Power Spectrum"] ("Item Names")
        w144 = "" ("Process States")
        # "Initialize the User Interface, here.\n(this is called automatically, by the Macro: Init)"
        n55 = call <userlib>:"User Library__ogtk.vi"() -> ("User Library (+ Relative)"=w139:path)  [unwired: 1 in]
        n56 = Build Path(base path=w139, name or relative path="LevyLab\\XY Utilities\\subVIs") -> (appended path=w138:path)
        n57 = local write "Process Queue"(w144) -> ()
        n58 = local write "Processed States"(w144) -> ()
        n59 = List Folder(path=w138) -> (filenames=w141:string[])  [unwired: 3 in, 3 out]
        n60 = local write "Graphs Tab Control"(enum32{"Data", "Intensity/Linecuts"}."Data" ("Graphs Tab Control")) -> ()
        n61 = local write "Tab Control"(enum32{"Page 1", "Page 2"}."Page 1" ("Tab Control")) -> ()
        n62 = property on="Available States" class="LstBox (strict)"("Val(Sgnl)"=-1 ("Value (Signaling)"), "Item Names"=w141) -> ()  [unwired: 2 in, 2 out]
        n63 = call <userlib>:"Fit VI window to Content__ogtk.vi"("error in (no error)"=w143) -> ("error out"=w142:errorcluster)  [unwired: 5 in, 1 out]
        n64 = call <vilib>:"Add State(s) to Queue__JKI_lib_State_Machine.vi"("State(s) in (\"\")"=w150) -> ("States Out"=w149:string)  [unwired: 14 in]
      }
      frame "UI: Cursor Set" {
        # "Argument"
        # "Set and Unset Cursor Busy.\n(Usage: \"UI: Cursor Set >> Busy|Idle\")"
        n65 = case shown="\"Idle\", Default" w151 {
          tunnel: w153 -> [w158 w160]
          tunnel: [w157 w159] -> w152
          frame "Idle", Default {
            n66 = call <vilib>:"Unset Busy.vi"("error in (no error)"=w158) -> ("error out"=w157:errorcluster)  [unwired: 10 in]
          }
          frame "Busy" {
            n67 = call <vilib>:"Set Busy.vi"("error in (no error)"=w160) -> ("error out"=w159:errorcluster)  [unwired: 9 in, 1 out]
          }
        }
        n68 = call <vilib>:"Add State(s) to Queue__JKI_lib_State_Machine.vi"("State(s) in (\"\")"=w156) -> ("States Out"=w155:string)  [unwired: 14 in]
      }
      frame "UI: Front Panel State" {
        # "Argument"
        # "Set Front Panel Open or Closed\n(Usage: \"UI: Front Panel State >> Open|Close\")"
        n69 = Unbundle By Name(w163) -> ("Core.Current VI Reference"=w162:refnum<vi>)
        n70 = case shown="\"Maximize\", \"Maximized\"" w161 {
          tunnel: w165 -> [w173 w188 w199 w212 w225]
          tunnel: [w175 w189 w201 w214 w227] -> w164
          tunnel: w162 -> [w174 w186 w200 w213 w226]
          frame "Open", "Standard", Default {
            w168 = T2."Standard" ("State")
            n71 = property class="VI"(reference=w174, error in=w173) -> (reference out=w171:refnum<vi>, error out=w172:errorcluster, "FP.State"=w170:T2)
            n72 = Not Equal?(x=w170, y=w168) -> (x != y?=w169:bool)
            n73 = case shown="True" w169 {
              tunnel: [w179 w181] -> w175
              tunnel: w172 -> [w178 w181]
              tunnel: w171 -> [w177 _]
              tunnel: w168 -> [w176 _]
              frame True {
                n74 = invoke class="VI" method="FP.Open"(reference=w177, error in=w178, "Activate"=TRUE, "State"=w176) -> (error out=w179:errorcluster)  [unwired: 1 in, 4 out]
              }
              frame False {
              }
            }
          }
          frame "Close", "Closed" {
            n75 = property class="VI"(reference=w186, error in=w188) -> (reference out=w185:refnum<vi>, error out=w187:errorcluster, "FP.State"=w183:T2)
            n76 = Not Equal?(x=w183, y=T2."Closed" ("Front Panel Window:State")) -> (x != y?=w182:bool)
            n77 = case shown="True" w182 {
              tunnel: [w190 w193] -> w189
              tunnel: w187 -> [w190 w192]
              tunnel: w185 -> [_ w191]
              frame False {
              }
              frame True {
                n78 = invoke class="VI" method="FP.Close"(reference=w191, error in=w192) -> (error out=w193:errorcluster)  [unwired: 1 in, 2 out]
              }
            }
          }
          frame "Hidden", "Hide" {
            w194 = T2."Hidden" ("State")
            n79 = property class="VI"(reference=w200, error in=w199) -> (reference out=w197:refnum<vi>, error out=w198:errorcluster, "FP.State"=w196:T2)
            n80 = Not Equal?(x=w196, y=w194) -> (x != y?=w195:bool)
            n81 = case shown="True" w195 {
              tunnel: [w205 w206] -> w201
              tunnel: w198 -> [w204 w206]
              tunnel: w197 -> [w203 _]
              tunnel: w194 -> [w202 _]
              frame True {
                n82 = invoke class="VI" method="FP.Open"(reference=w203, error in=w204, "State"=w202) -> (error out=w205:errorcluster)  [unwired: 2 in, 4 out]
              }
              frame False {
              }
            }
          }
          frame "Minimize", "Minimized" {
            w207 = T2."Minimized" ("State")
            n83 = property class="VI"(reference=w213, error in=w212) -> (reference out=w210:refnum<vi>, error out=w211:errorcluster, "FP.State"=w209:T2)
            n84 = Not Equal?(x=w209, y=w207) -> (x != y?=w208:bool)
            n85 = case shown="True" w208 {
              tunnel: [w218 w219] -> w214
              tunnel: w211 -> [w217 w219]
              tunnel: w210 -> [w216 _]
              tunnel: w207 -> [w215 _]
              frame True {
                n86 = invoke class="VI" method="FP.Open"(reference=w216, error in=w217, "State"=w215) -> (error out=w218:errorcluster)  [unwired: 2 in, 4 out]
              }
              frame False {
              }
            }
          }
          frame "Maximize", "Maximized" {
            w220 = T2."Maximized" ("State")
            n87 = property class="VI"(reference=w226, error in=w225) -> (reference out=w223:refnum<vi>, error out=w224:errorcluster, "FP.State"=w222:T2)
            n88 = Not Equal?(x=w222, y=w220) -> (x != y?=w221:bool)
            n89 = case shown="True" w221 {
              tunnel: [w231 w232] -> w227
              tunnel: w224 -> [w230 w232]
              tunnel: w223 -> [w229 _]
              tunnel: w220 -> [w228 _]
              frame True {
                n90 = invoke class="VI" method="FP.Open"(reference=w229, error in=w230, "State"=w228) -> (error out=w231:errorcluster)  [unwired: 2 in, 4 out]
              }
              frame False {
              }
            }
          }
        }
        n91 = call <vilib>:"Add State(s) to Queue__JKI_lib_State_Machine.vi"("State(s) in (\"\")"=w167) -> ("States Out"=w166:string)  [unwired: 14 in]
      }
      frame "---------- Macro ----------" {
        # "Do not put any code in this frame.\n(It is a separator no-op. You can make a copy of this frame to create a new Macro frame)"
        n92 = call <vilib>:"Add State(s) to Queue__JKI_lib_State_Machine.vi"("State(s) in (\"\")"=w236) -> ("States Out"=w235:string)  [unwired: 14 in]
      }
      frame "Macro: Initialize" {
        # "Initialization Macro\n(This is called once, when the VI starts)"
        n93 = call <vilib>:"Add State(s) to Queue__JKI_lib_State_Machine.vi"("State(s) in Front (\"\")"="Data: Initialize\nInitialize Core Data\nUI: Initialize\nUI: Front Panel State >> Open\nGraph: Initialize References 1\nGraph: Initialize References 2", "State(s) in (\"\")"=w241) -> ("States Out"=w240:string)  [unwired: 13 in]
      }
      frame "Macro: Exit" {
        # "Exit Macro\n(This is called once, when the VI exits)"
        n94 = Unbundle By Name(w248) -> ("Core.Close Panel on Exit?"=w247:bool)
        n95 = Select(t="UI: Front Panel State >> Close", s=w247, f="") -> (s? t:f=w244:string)
        n96 = call <vilib>:"Add State(s) to Queue__JKI_lib_State_Machine.vi"("State(s) in (\"\")"=w244, "State(s) at Back (\"\")"="Graph: Clear\nData: Cleanup\nExit") -> ("States Out"=w242:string)  [unwired: 13 in]
        n97 = call <vilib>:"Add State(s) to Queue__JKI_lib_State_Machine.vi"("State(s) in Front (\"\")"=w242, "State(s) in (\"\")"=w251) -> ("States Out"=w250:string)  [unwired: 13 in]
      }
      frame "Macro: Process" {
        # "XY: Add\nXY: Subtract\nXY: Multiply\nXY: Divide\nXY: Sort\nXY: Swap\nXY: Reverse\nXY: Subset\nXY: Derivative\nXY: Interpolate\nXY: FFT Spectrum\nXY: FFT Power Spectrum"
        # "Do not put any code in this frame.\n(It is a separator no-op. You can make a copy of this frame to create a new Macro frame)"
        n98 = call <vilib>:"Build State String with Arguments__JKI_lib_State_Machine.vi"("Arguments (\"\")"="Process Queue", "State"="XY: VI" ("State(s) in Front (\"\")")) -> ("State with Arguments"=w252:string)  [unwired: 4 in]
        n99 = call <vilib>:"Add State(s) to Queue__JKI_lib_State_Machine.vi"("State(s) in Front (\"\")"="UI: Cursor Set >> Busy\nFile: Load\nGraph: Initialize Graphs" ("State(s) in Front (\"\")"), "State(s) in (\"\")"=w252, "State(s) at Back (\"\")"="Graph: Update Graphs\nUI: Cursor Set >> Idle " ("State(s) in Front (\"\")")) -> ("States Out"=w255:string)  [unwired: 12 in]
        "Processed States" <- w255
        n100 = call <vilib>:"Add State(s) to Queue__JKI_lib_State_Machine.vi"("State(s) in Front (\"\")"=w255, "State(s) in (\"\")"=w261) -> ("States Out"=w260:string)  [unwired: 13 in]
      }
      frame "---------- Graph ----------" {
        # "Do not put any code in this frame.\n(It is a separator no-op. You can make a copy of this frame to create a new Macro frame)"
        n101 = call <vilib>:"Add State(s) to Queue__JKI_lib_State_Machine.vi"("State(s) in (\"\")"=w265) -> ("States Out"=w264:string)  [unwired: 14 in]
      }
      frame "Graph: Controls" {
        # "Do not put any code in this frame.\n(It is a separator no-op. You can make a copy of this frame to create a new Macro frame)"
        n102 = call <vilib>:"Add State(s) to Queue__JKI_lib_State_Machine.vi"("State(s) in (\"\")"=w269) -> ("States Out"=w268:string)  [unwired: 14 in]
      }
      frame "Graph: Initialize References 1" {
        # "Do not put any code in this frame.\n(It is a separator no-op. You can make a copy of this frame to create a new Data frame)"
        n103 = control-ref of="XY Graph: Unprocessed"() -> (w280:refnum<vi>)
        n104 = control-ref of="Data Intensity"() -> (w275:refnum<vi>)
        n105 = control-ref of="XY Graph: Processed"() -> (w274:refnum<vi>)
        n106 = call <userlib>:"Write Intensity Graph ref.vi"("error in (no error)"=w273, "Intensity Graph"=w275) -> ("error out"=w281:errorcluster, "graph_utilities out"=w279:refnum<class "graph_utilities.lvclass">)  [unwired: 8 in]
        n107 = call <userlib>:"Write Intensity Graph ref.vi"("error in (no error)"=w273, "Intensity Graph"=w275) -> ("error out"=w276:errorcluster, "graph_utilities out"=w271:refnum<class "graph_utilities.lvclass">)  [unwired: 8 in]
        n108 = call <userlib>:"Write XY Graph ref.vi"("error in (no error)"=w281, "XY Graph"=w280, "graph_utilities in"=w279) -> ("error out"=w277:errorcluster, "graph_utilities out"=w278:refnum<class "graph_utilities.lvclass">)  [unwired: 7 in]
        n109 = call <userlib>:"Write XY Graph ref.vi"("error in (no error)"=w276, "XY Graph"=w274, "graph_utilities in"=w271) -> ("error out"=w272:errorcluster, "graph_utilities out"=w270:refnum<class "graph_utilities.lvclass">)  [unwired: 7 in]
        n110 = Bundle By Name(cluster=w284, "Graph.Data: Unprocessed"=w278, "Graph.Data: Processed"=w270) -> (w283:T5)
        n111 = Merge Errors(w277, w272) -> (w282:errorcluster)
        n112 = call <vilib>:"Add State(s) to Queue__JKI_lib_State_Machine.vi"("State(s) in (\"\")"=w286) -> ("States Out"=w285:string)  [unwired: 14 in]
      }
      frame "Graph: Initialize References 2" {
        # "Do not put any code in this frame.\n(It is a separator no-op. You can make a copy of this frame to create a new Data frame)"
        n113 = control-ref of="Data Vertical"() -> (w306:refnum<vi>)
        n114 = control-ref of="Data Horizontal"() -> (w300:refnum<vi>)
        n115 = control-ref of="Diff Vertical"() -> (w305:refnum<vi>)
        n116 = control-ref of="Diff Horizontal"() -> (w303:refnum<vi>)
        n117 = control-ref of="Data Intensity"() -> (w288:refnum<vi>)
        n118 = control-ref of="Diff Intensity"() -> (w298:refnum<vi>)
        n119 = call <userlib>:"Write Intensity Graph ref.vi"("error in (no error)"=w287, "Intensity Graph (Control)"=w288, "Intensity Graph"=w288) -> ("error out"=w299:errorcluster, "graph_utilities out"=w301:refnum<class "graph_utilities.lvclass">)  [unwired: 7 in]
        n120 = call <userlib>:"Write Intensity Graph ref.vi"("error in (no error)"=w287, "Intensity Graph (Control)"=w288, "Intensity Graph"=w298) -> ("error out"=w302:errorcluster, "graph_utilities out"=w304:refnum<class "graph_utilities.lvclass">)  [unwired: 7 in]
        n121 = call <userlib>:"Write XY Graph ref.vi"("error in (no error)"=w299, "XY Graph"=w300, "graph_utilities in"=w301) -> ("error out"=w296:errorcluster, "graph_utilities out"=w291:refnum<class "graph_utilities.lvclass">)  [unwired: 7 in]
        n122 = call <userlib>:"Write XY Graph ref.vi"("error in (no error)"=w302, "XY Graph"=w303, "graph_utilities in"=w304) -> ("error out"=w297:errorcluster, "graph_utilities out"=w289:refnum<class "graph_utilities.lvclass">)  [unwired: 7 in]
        n123 = call <userlib>:"Write XY Graph ref.vi"("error in (no error)"=w296, "XY Graph"=w306, "graph_utilities in"=w301) -> ("error out"=w295:errorcluster, "graph_utilities out"=w292:refnum<class "graph_utilities.lvclass">)  [unwired: 7 in]
        n124 = call <userlib>:"Write XY Graph ref.vi"("error in (no error)"=w297, "XY Graph"=w305, "graph_utilities in"=w304) -> ("error out"=w294:errorcluster, "graph_utilities out"=w290:refnum<class "graph_utilities.lvclass">)  [unwired: 7 in]
        n125 = Bundle By Name(cluster=w308, "Graph.Data: Intensity/Vertical"=w292, "Graph.Data: Intensity/Horizontal"=w291, "Graph.Differential: Intensity/Vertical"=w290, "Graph.Differential: Intensity/Horizontal"=w289) -> (w307:T5)
        n126 = Merge Errors(w295, w294) -> (w293:errorcluster)
        n127 = call <vilib>:"Add State(s) to Queue__JKI_lib_State_Machine.vi"("State(s) in (\"\")"=w310) -> ("States Out"=w309:string)  [unwired: 14 in]
      }
      frame "Graph: Initialize Graphs" {
        # "Do not put any code in this frame.\n(It is a separator no-op. You can make a copy of this frame to create a new Macro frame)"
        n128 = Unbundle By Name(w315) -> ("Graph.Data: Unprocessed"=w318:refnum<class "graph_utilities.lvclass">, "XY Data (unprocessed)"=w313:cluster{"Intensity Data":dbl[], "Array":dbl[]}[], "Parameter"=w312:dbl[])
        n129 = call-poly <userlib>:"Set XY Graph Value.vi"("error in (no error)"=w314, "Value"=w313, "graph_utilities in"=w318) -> ("error out"=w317:errorcluster, "graph_utilities out"=w316:refnum<class "graph_utilities.lvclass">)  [unwired: 7 in]
        n130 = call <userlib>:"XY Graph to Intensity Graph.vi"("error in (no error)"=w317, "Y Scale"=w312, "graph_utilities in"=w316) -> ("error out"=w311:errorcluster)  [unwired: 7 in, 1 out]
        n131 = call <vilib>:"Add State(s) to Queue__JKI_lib_State_Machine.vi"("State(s) in (\"\")"=w320) -> ("States Out"=w319:string)  [unwired: 14 in]
      }
      frame "Graph: Update Graphs" {
        # "Do not put any code in this frame.\n(It is a separator no-op. You can make a copy of this frame to create a new UI frame)"
        n132 = Unbundle By Name(w328) -> ("Graph.Data: Processed"=w327:refnum<class "graph_utilities.lvclass">, "XY Data (processed 1)"=w326:cluster{"Intensity Data":dbl[], "Array":dbl[]}[], "Parameter"=w323:dbl[])
        n133 = call-poly <userlib>:"Set XY Graph Value.vi"("error in (no error)"=w325, "Value"=w326, "graph_utilities in"=w327) -> ("error out"=w322:errorcluster, "graph_utilities out"=w324:refnum<class "graph_utilities.lvclass">)  [unwired: 7 in]
        n134 = call <userlib>:"XY Graph to Intensity Graph.vi"("error in (no error)"=w322, "Y Scale"=w323, "graph_utilities in"=w324) -> ("error out"=w321:errorcluster)  [unwired: 7 in, 1 out]
        n135 = call <vilib>:"Add State(s) to Queue__JKI_lib_State_Machine.vi"("State(s) in (\"\")"=w330) -> ("States Out"=w329:string)  [unwired: 14 in]
      }
      frame "Graph: Clear" {
        w331 = cluster{dbl[], dbl[]}[] [] ("Value")
        w334 = dbl[][] [] ("Value")
        # "Do not put any code in this frame.\n(It is a separator no-op. You can make a copy of this frame to create a new Macro frame)"
        n136 = Unbundle By Name(w351) -> ("Graph.Data: Unprocessed"=w335:refnum<class "graph_utilities.lvclass">, "Graph.Data: Processed"=w350:refnum<class "graph_utilities.lvclass">, "Graph.Data: Intensity/Vertical"=w344:refnum<class "graph_utilities.lvclass">, "Graph.Data: Intensity/Horizontal"=w343:refnum<class "graph_utilities.lvclass">, "Graph.Differential: Intensity/Vertical"=w342:refnum<class "graph_utilities.lvclass">, "Graph.Differential: Intensity/Horizontal"=w341:refnum<class "graph_utilities.lvclass">)
        n137 = call <userlib>:"Set Intensity Graph Value.vi"("Value"=w334, "graph_utilities in"=w335) -> ("error out"=w332:errorcluster, "graph_utilities out"=w333:refnum<class "graph_utilities.lvclass">)  [unwired: 8 in]
        n138 = call <userlib>:"Set Intensity Graph Value.vi"("Value"=w334, "graph_utilities in"=w350) -> ("error out"=w340:errorcluster, "graph_utilities out"=w349:refnum<class "graph_utilities.lvclass">)  [unwired: 8 in]
        n139 = call <userlib>:"Set Intensity Graph Value.vi"("Value"=w334, "graph_utilities in"=w343) -> ("error out"=w338:errorcluster, "graph_utilities out"=w347:refnum<class "graph_utilities.lvclass">)  [unwired: 8 in]
        n140 = call <userlib>:"Set Intensity Graph Value.vi"("Value"=w334, "graph_utilities in"=w344) -> ("error out"=w339:errorcluster, "graph_utilities out"=w348:refnum<class "graph_utilities.lvclass">)  [unwired: 8 in]
        n141 = call <userlib>:"Set Intensity Graph Value.vi"("Value"=w334, "graph_utilities in"=w342) -> ("error out"=w337:errorcluster, "graph_utilities out"=w346:refnum<class "graph_utilities.lvclass">)  [unwired: 8 in]
        n142 = call <userlib>:"Set Intensity Graph Value.vi"("Value"=w334, "graph_utilities in"=w341) -> ("error out"=w336:errorcluster, "graph_utilities out"=w345:refnum<class "graph_utilities.lvclass">)  [unwired: 8 in]
        n143 = call-poly <userlib>:"Set XY Graph Value.vi"("error in (no error)"=w332, "Value"=w331, "graph_utilities in"=w333) -> ()  [unwired: 7 in, 2 out]
        n144 = call-poly <userlib>:"Set XY Graph Value.vi"("error in (no error)"=w340, "Value"=w331, "graph_utilities in"=w349) -> ()  [unwired: 7 in, 2 out]
        n145 = call-poly <userlib>:"Set XY Graph Value.vi"("error in (no error)"=w338, "Value"=w331, "graph_utilities in"=w347) -> ()  [unwired: 7 in, 2 out]
        n146 = call-poly <userlib>:"Set XY Graph Value.vi"("error in (no error)"=w339, "Value"=w331, "graph_utilities in"=w348) -> ()  [unwired: 7 in, 2 out]
        n147 = call-poly <userlib>:"Set XY Graph Value.vi"("error in (no error)"=w337, "Value"=w331, "graph_utilities in"=w346) -> ()  [unwired: 7 in, 2 out]
        n148 = call-poly <userlib>:"Set XY Graph Value.vi"("error in (no error)"=w336, "Value"=w331, "graph_utilities in"=w345) -> ()  [unwired: 7 in, 2 out]
        n149 = local write "XY Graph: Antisymmetric"(w331) -> ()
        n150 = local write "XY Graph: Symmetric"(w331) -> ()
        n151 = call <vilib>:"Add State(s) to Queue__JKI_lib_State_Machine.vi"("State(s) in (\"\")"=w354) -> ("States Out"=w353:string)  [unwired: 14 in]
      }
      frame "Graph: Linecut" {
        # "Do not put any code in this frame.\n(It is a separator no-op. You can make a copy of this frame to create a new Macro frame)"
        n152 = Unbundle By Name(w368) -> ("Graph.Data: Intensity/Vertical"=w367:refnum<class "graph_utilities.lvclass">, "Graph.Data: Intensity/Horizontal"=w366:refnum<class "graph_utilities.lvclass">, "Graph.Differential: Intensity/Vertical"=w365:refnum<class "graph_utilities.lvclass">, "Graph.Differential: Intensity/Horizontal"=w364:refnum<class "graph_utilities.lvclass">)
        n153 = call <userlib>:"Intensity Graph Linecut (Vertical).vi"("error in (no error)"=w361, "width (vertical)"="width (vertical)", "graph_utilities in"=w367) -> ("error out"=w362:errorcluster)  [unwired: 7 in, 1 out]
        n154 = call <userlib>:"Intensity Graph Linecut (Horizontal).vi"("error in (no error)"=w362, "width (horizontal)"="width (horizontal)", "graph_utilities in"=w366) -> ("error out"=w363:errorcluster)  [unwired: 7 in, 1 out]
        n155 = call <userlib>:"Intensity Graph Linecut (Vertical).vi"("error in (no error)"=w363, "width (vertical)"="width (vertical) 2", "graph_utilities in"=w365) -> ("error out"=w360:errorcluster)  [unwired: 7 in, 1 out]
        n156 = call <userlib>:"Intensity Graph Linecut (Horizontal).vi"("error in (no error)"=w360, "width (horizontal)"="width (horizontal) 2", "graph_utilities in"=w364) -> ("error out"=w359:errorcluster)  [unwired: 7 in, 1 out]
        n157 = call <vilib>:"Add State(s) to Queue__JKI_lib_State_Machine.vi"("State(s) in (\"\")"=w370) -> ("States Out"=w369:string)  [unwired: 14 in]
      }
      frame "---------- File ----------" {
        # "Do not put any code in this frame.\n(It is a separator no-op. You can make a copy of this frame to create a new Macro frame)"
        n158 = call <vilib>:"Add State(s) to Queue__JKI_lib_State_Machine.vi"("State(s) in (\"\")"=w374) -> ("States Out"=w373:string)  [unwired: 14 in]
      }
      frame "File: Load" {
        (unwired) dbl[] [-9.0, -8.75, -8.5, -8.25, -8.0, -7.75, -7.5, -7.25, -7.0, -6.75, -6.5, -6.25, -6.0, -5.75, -5.5, -5.25, -5.0, -4.75, -4.5, -4.25, -4.0, -3.75, -3.5, -3.25, -3.0, -2.75, -2.5, -2.25, -2.0, -1.75, -1.5, -1.25, -1.0, -0.75, -0.5, -0.25, 0.0, 0.25, 0.5, 0.75, 1.0, 1.25, 1.5, 1.75, 2.0, 2.25, 2.5, 2.75, 3.0, 3.25, 3.5, 3.75, 4.0, 4.25, 4.5, 4.75, 5.0, 5.25, 5.5, 5.75, 6.0, 6.25, 6.5, 6.75, 7.0, 7.25, 7.5, 7.75, 8.0, 8.25, 8.5, 8.75, 9.0] ("X")
        (unwired) cluster{"Intensity Data":dbl[], "Array":dbl[]}[] [{"Intensity Data"=[0.0, 0.004, 0.008, 0.012, 0.016, 0.02, 0.024, 0.028, 0.032, 0.036000000000000004, 0.04, 0.044, 0.048, 0.052000000000000005, 0.056, 0.06, 0.064, 0.068, 0.07200000000000001, 0.076, 0.08, 0.084, 0.088, 0.092, 0.096, 0.1, 0.10400000000000001, 0.108, 0.112, 0.116, 0.12, 0.124, 0.128, 0.132, 0.136, 0.14, 0.14400000000000002, 0.148, 0.152, 0.156, 0.16, 0.164, 0.168, 0.17200000000000001, 0.176, 0.18, 0.184, 0.188, 0.192, 0.196, 0.2, 0.20400000000000001, 0.20800000000000002, 0.212, 0.216, 0.22, 0.224, 0.228, 0.232, 0.23600000000000002, 0.24, 0.244, 0.248, 0.252, 0.256, 0.26, 0.264, 0.268, 0.272, 0.276, 0.28, 0.28400000000000003, 0.28800000000000003, 0.292, 0.296, 0.3, 0.304, 0.308, 0.312, 0.316, 0.32, 0.324, 0.328, 0.332, 0.336, 0.34, 0.34400000000000003, 0.34800000000000003, 0.352, 0.356, 0.36, 0.364, 0.368, 0.372, 0.376, 0.38, 0.384, 0.388, 0.392, 0.396, 0.4, 0.404, 0.40800000000000003, 0.41200000000000003, 0.41600000000000004, 0.42, 0.424, 0.428, 0.432, 0.436, 0.44, 0.444, 0.448, 0.452, 0.456, 0.46, 0.464, 0.468, 0.47200000000000003, 0.47600000000000003, 0.48, 0.484, 0.488, 0.492, 0.496, 0.5, 0.504, 0.508, 0.512, 0.516, 0.52, 0.524, 0.528, 0.532, 0.536, 0.54, 0.544, 0.548, 0.552, 0.556, 0.56, 0.5640000000000001, 0.5680000000000001, 0.5720000000000001, 0.5760000000000001, 0.58, 0.584, 0.588, 0.592, 0.596, 0.6, 0.604, 0.608, 0.612, 0.616, 0.62, 0.624, 0.628, 0.632, 0.636, 0.64, 0.644, 0.648, 0.652, 0.656, 0.66, 0.664, 0.668, 0.672, 0.676, 0.68, 0.684, 0.6880000000000001, 0.6920000000000001, 0.6960000000000001, 0.7000000000000001, 0.704, 0.708, 0.712, 0.716, 0.72, 0.724, 0.728, 0.732, 0.736, 0.74, 0.744, 0.748, 0.752, 0.756, 0.76, 0.764, 0.768, 0.772, 0.776, 0.78, 0.784, 0.788, 0.792, 0.796, 0.8, 0.804, 0.808, 0.812, 0.8160000000000001, 0.8200000000000001, 0.8240000000000001, 0.8280000000000001, 0.8320000000000001, 0.836, 0.84, 0.844, 0.848, 0.852, 0.856, 0.86, 0.864, 0.868, 0.872, 0.876, 0.88], "Array"=[1.68063e-07, 1.37198e-07, 8.79687e-08, 1.06463e-07, 1.07999e-07, 1.50443e-07, 1.6136e-07, 1.60216e-07, 1.51628e-07, 1.62347e-07, 2.24052e-07, 2.12498e-07, 1.69888e-07, 2.07771e-07, 2.10504e-07, 1.16164e-07, 1.03648e-07, 1.88353e-07, 2.52956e-07, 1.81322e-07, 1.3598e-07, 1.93502e-07, 3.06623e-07, 1.81397e-07, 1.56136e-07, 7.65771e-08, 1.0323e-07, 2.25052e-07, 2.18994e-07, 1.48687e-07, 1.23465e-07, 1.94812e-07, 8.89733e-08, 1.01215e-07, 1.91375e-07, 1.83998e-07, 1.70281e-07, 2.66741e-07, 1.84557e-07, 1.35922e-07, 1.53284e-07, 1.28241e-07, 1.84801e-07, 1.04068e-07, 8.03285e-08, 1.04402e-07, 8.12206e-08, 5.15301e-08, 2.02427e-07, 1.78907e-07, 1.0348e-07, 8.96397e-08, 1.49064e-07, 2.10614e-07, 1.94321e-07, 1.23458e-07, 2.49381e-08, 1.85551e-07, 1.98644e-07, 2.30779e-07, 3.77495e-07, 6.72036e-07, 1.17947e-06, 1.75588e-06, 2.53801e-06, 3.50995e-06, 4.10398e-06, 4.4421e-06, 4.54957e-06, 4.46684e-06, 4.29614e-06, 4.03689e-06, 3.7785e-06, 3.52652e-06, 3.3015e-06, 3.0176e-06, 2.73351e-06, 2.48081e-06, 2.28944e-06, 2.06704e-06, 1.80961e-06, 1.62787e-06, 1.44499e-06, 1.27341e-06, 1.12003e-06, 1.00442e-06, 8.63595e-07, 7.29893e-07, 6.0347e-07, 5.41881e-07, 4.90755e-07, 4.14075e-07, 3.64346e-07, 3.41478e-07, 3.11551e-07, 2.93279e-07, 3.09014e-07, 3.23829e-07, 3.14767e-07, 3.13298e-07, 3.2943e-07, 3.73559e-07, 3.85052e-07, 4.12776e-07, 4.52513e-07, 4.63779e-07, 5.00565e-07, 5.25226e-07, 5.28226e-07, 5.09122e-07, 4.69838e-07, 4.77525e-07, 4.87608e-07, 4.64681e-07, 4.29366e-07, 4.10075e-07, 3.911e-07, 3.53091e-07, 3.11529e-07, 2.80052e-07, 2.48962e-07, 2.2069e-07, 2.00389e-07, 1.80056e-07, 1.71025e-07, 1.52747e-07, 1.20455e-07, 1.10317e-07, 1.22804e-07, 1.19285e-07, 1.05556e-07, 1.00514e-07, 1.16004e-07, 1.33715e-07, 1.48638e-07, 1.67858e-07, 1.60768e-07, 1.72191e-07, 1.90163e-07, 2.12957e-07, 2.27031e-07, 2.42395e-07, 2.5957e-07, 2.75457e-07, 2.81378e-07, 2.87991e-07, 2.8598e-07, 2.99029e-07, 3.10983e-07, 2.98582e-07, 2.92597e-07, 2.96466e-07, 2.75316e-07, 2.60924e-07, 2.73094e-07, 2.76228e-07, 2.69051e-07, 2.49348e-07, 2.40239e-07, 2.38694e-07, 2.46997e-07, 2.3754e-07, 2.31936e-07, 2.37921e-07, 2.4129e-07, 2.36577e-07, 2.27175e-07, 2.23179e-07, 2.32753e-07, 2.22017e-07, 2.21659e-07, 2.35338e-07, 2.45551e-07, 2.48375e-07, 2.61624e-07, 2.68417e-07, 2.63606e-07, 2.83272e-07, 2.96328e-07, 2.89196e-07, 2.96568e-07, 3.03707e-07, 3.06523e-07, 3.1915e-07, 3.12655e-07, 2.95357e-07, 2.95008e-07, 2.98448e-07, 3.09012e-07, 3.01923e-07, 2.96206e-07, 3.10244e-07, 3.04155e-07, 2.92192e-07, 2.85057e-07, 2.82269e-07, 2.90168e-07, 2.75276e-07, 2.42554e-07, 2.36848e-07, 2.39448e-07, 2.14838e-07, 2.06682e-07, 2.0462e-07, 1.85893e-07, 1.77192e-07, 1.71389e-07, 1.56772e-07, 1.51419e-07, 1.47796e-07, 1.53989e-07, 1.38128e-07, 1.40478e-07, 1.52301e-07, 1.42379e-07, 1.31716e-07, 1.3604e-07, 1.51662e-07, 1.43388e-07, 1.35586e-07, 1.45146e-07]}, ...(73 in all)] ("Vertical")
        # "Add code here for loading your data from disk"
        # "File: Load\n(Add code here for loading your data)"
        n159 = Unbundle By Name("Channels") -> ("X"=w379:string, "Y"=w378:string, "N"=w377:string)
        n160 = for {
          N: "Numeric" -> [_]
          tunnel: "File or Folder Path" -> [w392]
          tunnel: [w402] -> w382 mode=indexing
          tunnel: [w396] -> w381 mode=indexing
          tunnel: [w395] -> _
          tunnel: w379 -> [w391]
          tunnel: w378 -> [w389]
          tunnel: w377 -> [w390]
          i -> [w388]
          n161 = call <userlib>:"Read TDMS Wave 1D.vi"("Append Index"=w388, "channel name(s) in"=w391, "path"=w392) -> ("error out"=w401:errorcluster, "data"=w393:dbl[], "file path out"=w400:path)  [unwired: 6 in]
          n162 = call <userlib>:"Read TDMS Wave 1D.vi"("Append Index"=w388, "error in (no error)"=w401, "channel name(s) in"=w389, "path"=w400) -> ("error out"=w399:errorcluster, "data"=w394:dbl[], "file path out"=w398:path)  [unwired: 5 in]
          n163 = call <userlib>:"Read TDMS Wave 1D.vi"("Append Index"=w388, "error in (no error)"=w399, "channel name(s) in"=w390, "path"=w398) -> ("error out"=w395:errorcluster, "data"=w397:dbl[])  [unwired: 5 in, 1 out]
          n164 = Index Array(array=w397) -> (element=w396:dbl)  [unwired: 1 in]
          n165 = Bundle("data"=w394, "data"=w393) -> (w402:cluster{"data":dbl[], "data":dbl[]})  [unwired: 1 in]
          "counter" <- w388
        }
        n166 = Bundle By Name(cluster=w384, "XY Data (unprocessed)"=w382, "XY Data (processed 1)"=w382, "XY Data (processed 2)"=w382, "Parameter"=w381) -> (w385:T5)
        n167 = call <vilib>:"Add State(s) to Queue__JKI_lib_State_Machine.vi"("State(s) in (\"\")"=w387) -> ("States Out"=w386:string)  [unwired: 14 in]
      }
      frame "---------- XY ----------" {
        # "Template Separator\n(You can make a copy of, or modify, this frame)"
        n168 = Unbundle By Name(w407) -> ("XY Data (processed 1)"=w408:cluster{"Intensity Data":dbl[], "Array":dbl[]}[])
        n169 = call-poly <userlib>:"Add.vi"("error in (no error)"=w404, "XY-data"=w408) -> ("error out"=w403:errorcluster, "XY-data out"=w405:cluster{"X-array":dbl[], "Y-array":dbl[]}[])  [unwired: 8 in]
        n170 = Bundle By Name(cluster=w407, "XY Data (processed 1)"=w405) -> (w406:T5)
        n171 = call <vilib>:"Add State(s) to Queue__JKI_lib_State_Machine.vi"("State(s) in (\"\")"=w410) -> ("States Out"=w409:string)  [unwired: 14 in]
      }
      frame "XY: VI Filter" {
        # "Template Separator\n(You can make a copy of, or modify, this frame)"
        n172 = disable-structure shown="Enabled" {
          disable-tunnel: w415 -> [w434 w436]
          disable-tunnel: [w433 w436] -> w414
          disable-tunnel: w413 -> [w429 _]
          disable-tunnel: w412 -> [w424 w435]
          disable-tunnel: [w420 w435] -> w411
          frame Disabled {
            n173 = Unbundle By Name(w434) -> ("XY Data (processed 1)"=w426:cluster{"Intensity Data":dbl[], "Array":dbl[]}[])
            n174 = call <userlib>:"User Library__ogtk.vi"() -> ("User Library (+ Relative)"=w431:path)  [unwired: 1 in]
            n175 = Build Path(base path=w431, name or relative path="LevyLab\\XY Utilities\\subVIs") -> (appended path=w430:path)
            n176 = Build Path(base path=w430, name or relative path=w429) -> (appended path=w428:path)
            n177 = Open VI Reference(type specifier VI Refnum (for type only)=refnum<vi> refnum, vi path=w428, error in (no error)=w424) -> (vi reference=w427:refnum<vi>, error out=w423:errorcluster)  [unwired: 3 in]
            n178 = local read "x"() -> (w419:dbl)
            n179 = call-by-ref "?"(reference=w427, error in=w423, "y (0)"=w419, "XY-data"=w426) -> (reference out=w422:refnum<vi>, error out=w421:errorcluster, "XY-data out"=w425:cluster{"X-array":dbl[], "Y-array":dbl[]}[])  [unwired: 8 in, 1 out]
            n180 = call-poly <userlib>:"Add.vi"() -> ()  [unwired: 10 in, 2 out]
            n181 = Close Reference(reference=w422, error in (no error)=w421) -> (error out=w420:errorcluster)
            n182 = Bundle By Name(cluster=w434, "XY Data (processed 1)"=w425) -> (w433:T5)
          }
          frame Enabled {
          }
        }
        n183 = call <vilib>:"Add State(s) to Queue__JKI_lib_State_Machine.vi"("State(s) in (\"\")"=w417) -> ("States Out"=w416:string)  [unwired: 14 in]
      }
      frame "XY: Add" {
        # "XY: Add\n(You can make a copy of, or modify, this frame)"
        n184 = Unbundle By Name(w443) -> ("XY Data (processed 1)"=w444:cluster{"Intensity Data":dbl[], "Array":dbl[]}[])
        n185 = call-poly <userlib>:"Add.vi"("error in (no error)"=w440, "y (0)"="y", "x (0)"="x", "XY-data"=w444) -> ("error out"=w439:errorcluster, "XY-data out"=w441:cluster{"X-array":dbl[], "Y-array":dbl[]}[])  [unwired: 6 in]
        n186 = Bundle By Name(cluster=w443, "XY Data (processed 1)"=w441) -> (w442:T5)
        n187 = call <vilib>:"Add State(s) to Queue__JKI_lib_State_Machine.vi"("State(s) in (\"\")"=w446) -> ("States Out"=w445:string)  [unwired: 14 in]
      }
      frame "XY: Subtract" {
        # "Template Separator\n(You can make a copy of, or modify, this frame)"
        n188 = Unbundle By Name(w453) -> ("XY Data (processed 1)"=w454:cluster{"Intensity Data":dbl[], "Array":dbl[]}[])
        n189 = local read "x"() -> (w447:dbl)
        n190 = local read "y"() -> (w448:dbl)
        n191 = call-poly <userlib>:"Subtract.vi"("error in (no error)"=w450, "y (0)"=w448, "x (0)"=w447, "XY-data"=w454) -> ("error out"=w449:errorcluster, "XY-data out"=w451:cluster{"X-array":dbl[], "Y-array":dbl[]}[])  [unwired: 6 in]
        n192 = Bundle By Name(cluster=w453, "XY Data (processed 1)"=w451) -> (w452:T5)
        n193 = call <vilib>:"Add State(s) to Queue__JKI_lib_State_Machine.vi"("State(s) in (\"\")"=w456) -> ("States Out"=w455:string)  [unwired: 14 in]
      }
      frame "XY: Multiply" {
        # "Template Separator\n(You can make a copy of, or modify, this frame)"
        n194 = Unbundle By Name(w463) -> ("XY Data (processed 1)"=w464:cluster{"Intensity Data":dbl[], "Array":dbl[]}[])
        n195 = local read "x"() -> (w458:dbl)
        n196 = local read "y"() -> (w457:dbl)
        n197 = call-poly <userlib>:"Multiply.vi"("error in (no error)"=w460, "y (1)"=w457, "x (1)"=w458, "XY-data"=w464) -> ("error out"=w459:errorcluster, "XY-data out"=w461:cluster{"X-array":dbl[], "Y-array":dbl[]}[])  [unwired: 6 in]
        n198 = Bundle By Name(cluster=w463, "XY Data (processed 1)"=w461) -> (w462:T5)
        n199 = call <vilib>:"Add State(s) to Queue__JKI_lib_State_Machine.vi"("State(s) in (\"\")"=w466) -> ("States Out"=w465:string)  [unwired: 14 in]
      }
      frame "XY: Square" {
        # "Template Separator\n(You can make a copy of, or modify, this frame)"
        n200 = Unbundle By Name(w471) -> ("XY Data (processed 1)"=w472:cluster{"Intensity Data":dbl[], "Array":dbl[]}[])
        n201 = call-poly <userlib>:"Square.vi"("error in (no error)"=w468, "XY-data"=w472) -> ("error out"=w467:errorcluster, "XY-data out"=w469:cluster{"X-array":dbl[], "Y-array":dbl[]}[])  [unwired: 8 in]
        n202 = Bundle By Name(cluster=w471, "XY Data (processed 1)"=w469) -> (w470:T5)
        n203 = call <vilib>:"Add State(s) to Queue__JKI_lib_State_Machine.vi"("State(s) in (\"\")"=w474) -> ("States Out"=w473:string)  [unwired: 14 in]
      }
      frame "XY: Divide" {
        # "Template Separator\n(You can make a copy of, or modify, this frame)"
        n204 = Unbundle By Name(w481) -> ("XY Data (processed 1)"=w482:cluster{"Intensity Data":dbl[], "Array":dbl[]}[])
        n205 = local read "x"() -> (w476:dbl)
        n206 = local read "y"() -> (w475:dbl)
        n207 = call-poly <userlib>:"Divide.vi"("error in (no error)"=w478, "y (1)"=w475, "x (1)"=w476, "XY-data"=w482) -> ("error out"=w477:errorcluster, "XY-data out"=w479:cluster{"X-array":dbl[], "Y-array":dbl[]}[])  [unwired: 6 in]
        n208 = Bundle By Name(cluster=w481, "XY Data (processed 1)"=w479) -> (w480:T5)
        n209 = call <vilib>:"Add State(s) to Queue__JKI_lib_State_Machine.vi"("State(s) in (\"\")"=w484) -> ("States Out"=w483:string)  [unwired: 14 in]
      }
      frame "XY: Sort" {
        # "Template Separator\n(You can make a copy of, or modify, this frame)"
        n210 = Unbundle By Name(w489) -> ("XY Data (processed 1)"=w490:cluster{"Intensity Data":dbl[], "Array":dbl[]}[])
        n211 = call-poly <userlib>:"Sort.vi"("error in (no error)"=w486, "XY-data"=w490) -> ("error out"=w485:errorcluster, "Sorted XY-data out"=w487:cluster{"X-array":dbl[], "Y-array":dbl[]}[])  [unwired: 8 in]
        n212 = Bundle By Name(cluster=w489, "XY Data (processed 1)"=w487) -> (w488:T5)
        n213 = call <vilib>:"Add State(s) to Queue__JKI_lib_State_Machine.vi"("State(s) in (\"\")"=w492) -> ("States Out"=w491:string)  [unwired: 14 in]
      }
      frame "XY: Swap" {
        # "Template Separator\n(You can make a copy of, or modify, this frame)"
        n214 = Unbundle By Name(w497) -> ("XY Data (processed 1)"=w498:cluster{"Intensity Data":dbl[], "Array":dbl[]}[])
        n215 = call-poly <userlib>:"Swap X and Y.vi"("error in (no error)"=w494, "XY-data"=w498) -> ("error out"=w493:errorcluster, "XY-data out"=w495:cluster{"X-array":dbl[], "Y-array":dbl[]}[])  [unwired: 8 in]
        n216 = Bundle By Name(cluster=w497, "XY Data (processed 1)"=w495) -> (w496:T5)
        n217 = call <vilib>:"Add State(s) to Queue__JKI_lib_State_Machine.vi"("State(s) in (\"\")"=w500) -> ("States Out"=w499:string)  [unwired: 14 in]
      }
      frame "XY: Reverse" {
        # "Template Separator\n(You can make a copy of, or modify, this frame)"
        n218 = Unbundle By Name(w505) -> ("XY Data (processed 1)"=w506:cluster{"Intensity Data":dbl[], "Array":dbl[]}[])
        n219 = call-poly <userlib>:"Reverse.vi"("error in (no error)"=w502, "XY-data"=w506) -> ("error out"=w501:errorcluster, "Reversed XY-data out"=w503:cluster{"X-array":dbl[], "Y-array":dbl[]}[])  [unwired: 8 in]
        n220 = Bundle By Name(cluster=w505, "XY Data (processed 1)"=w503) -> (w504:T5)
        n221 = call <vilib>:"Add State(s) to Queue__JKI_lib_State_Machine.vi"("State(s) in (\"\")"=w508) -> ("States Out"=w507:string)  [unwired: 14 in]
      }
      frame "XY: Subset" {
        # "Template Separator\n(You can make a copy of, or modify, this frame)"
        n222 = Unbundle By Name(w515) -> ("XY Data (processed 1)"=w516:cluster{"Intensity Data":dbl[], "Array":dbl[]}[])
        n223 = call-poly <userlib>:"Subset.vi"("error in (no error)"=w512, "Subset Method"="Method", "Subset Slider"="Subset Slider", "XY-data"=w516) -> ("error out"=w511:errorcluster, "Subset XY-data out"=w513:cluster{"X-array":dbl[], "Y-array":dbl[]}[])  [unwired: 6 in]
        n224 = Bundle By Name(cluster=w515, "XY Data (processed 1)"=w513) -> (w514:T5)
        n225 = call <vilib>:"Add State(s) to Queue__JKI_lib_State_Machine.vi"("State(s) in (\"\")"=w518) -> ("States Out"=w517:string)  [unwired: 14 in]
      }
      frame "XY: Derivative" {
        # "Template Separator\n(You can make a copy of, or modify, this frame)"
        n226 = Unbundle By Name(w526) -> ("XY Data (processed 1)"=w527:cluster{"Intensity Data":dbl[], "Array":dbl[]}[])
        n227 = call-poly <userlib>:"Derivative.vi"("Interval Units"="Interval Units", "error in (no error)"=w524, "Type"="Type", "Interval"="Interval", "XY-data"=w527) -> ("error out"=w523:errorcluster, "Differential out"=w519:cluster{"X-array":dbl[], "Y-array":dbl[]}[])  [unwired: 4 in, 1 out]
        n228 = Bundle By Name(cluster=w526, "XY Data (processed 1)"=w519) -> (w525:T5)
        n229 = call <vilib>:"Add State(s) to Queue__JKI_lib_State_Machine.vi"("State(s) in (\"\")"=w529) -> ("States Out"=w528:string)  [unwired: 14 in]
      }
      frame "XY: Interpolate" {
        # "Template Separator\n(You can make a copy of, or modify, this frame)"
        n230 = Unbundle By Name(w535) -> ("XY Data (processed 1)"=w536:cluster{"Intensity Data":dbl[], "Array":dbl[]}[])
        n231 = call-poly <userlib>:"Interpolate.vi"("error in (no error)"=w532, "Configure"="Configure", "XY-data"=w536) -> ("error out"=w531:errorcluster, "Interpolated XY-data out"=w533:cluster{"X-array":dbl[], "Y-array":dbl[]}[])  [unwired: 7 in]
        n232 = Bundle By Name(cluster=w535, "XY Data (processed 1)"=w533) -> (w534:T5)
        n233 = call <vilib>:"Add State(s) to Queue__JKI_lib_State_Machine.vi"("State(s) in (\"\")"=w538) -> ("States Out"=w537:string)  [unwired: 14 in]
      }
      frame "XY: FFT Spectrum" {
        # "Template Separator\n(You can make a copy of, or modify, this frame)"
        n234 = Unbundle By Name(w543) -> ("XY Data (processed 1)"=w544:cluster{"Intensity Data":dbl[], "Array":dbl[]}[])
        n235 = call-poly <userlib>:"FFT Spectrum.vi"("error in (no error)"=w540, "XY-data"=w544) -> ("error out"=w539:errorcluster, "XY-data out"=w541:cluster{"X-array":dbl[], "Y-array":dbl[]}[])  [unwired: 6 in, 2 out]
        n236 = Bundle By Name(cluster=w543, "XY Data (processed 1)"=w541) -> (w542:T5)
        n237 = call <vilib>:"Add State(s) to Queue__JKI_lib_State_Machine.vi"("State(s) in (\"\")"=w546) -> ("States Out"=w545:string)  [unwired: 14 in]
      }
      frame "XY: FFT Power Spectrum" {
        # "Template Separator\n(You can make a copy of, or modify, this frame)"
        n238 = Unbundle By Name(w551) -> ("XY Data (processed 1)"=w552:cluster{"Intensity Data":dbl[], "Array":dbl[]}[])
        n239 = call-poly <userlib>:"FFT Power Spectrum.vi"("error in (no error)"=w549, "XY-data"=w552) -> ("error out"=w548:errorcluster, "XY-data out"=w547:cluster{"X-array":dbl[], "Y-array":dbl[]}[])  [unwired: 7 in, 1 out]
        n240 = Bundle By Name(cluster=w551, "XY Data (processed 1)"=w547) -> (w550:T5)
        n241 = call <vilib>:"Add State(s) to Queue__JKI_lib_State_Machine.vi"("State(s) in (\"\")"=w554) -> ("States Out"=w553:string)  [unwired: 14 in]
      }
      frame "XY: Resample" {
        # "Template Separator\n(You can make a copy of, or modify, this frame)"
        n242 = Unbundle By Name(w559) -> ("XY Data (processed 1)"=w560:cluster{"Intensity Data":dbl[], "Array":dbl[]}[])
        n243 = call-poly <userlib>:"Resample.vi"("error in (no error)"=w556, "XY-data"=w560) -> ("error out"=w555:errorcluster, "Resampled XY-data out"=w557:cluster{"X-array":dbl[], "Y-array":dbl[]}[])  [unwired: 8 in]
        n244 = Bundle By Name(cluster=w559, "XY Data (processed 1)"=w557) -> (w558:T5)
        n245 = call <vilib>:"Add State(s) to Queue__JKI_lib_State_Machine.vi"("State(s) in (\"\")"=w562) -> ("States Out"=w561:string)  [unwired: 14 in]
      }
      frame "XY: Average" {
        # "Template Separator\n(You can make a copy of, or modify, this frame)"
        n246 = Unbundle By Name(w567) -> ("XY Data (processed 1)"=w568:cluster{"Intensity Data":dbl[], "Array":dbl[]}[])
        n247 = call <userlib>:"Average.vi"("error in (no error)"=w564, "XY-data"=w568) -> ("error out"=w563:errorcluster, "XY-data out"=w565:cluster{"X-array":dbl[], "Y-array":dbl[]}[])  [unwired: 7 in, 1 out]
        n248 = Bundle By Name(cluster=w567, "XY Data (processed 1)"=w565) -> (w566:T5)
        n249 = call <vilib>:"Add State(s) to Queue__JKI_lib_State_Machine.vi"("State(s) in (\"\")"=w570) -> ("States Out"=w569:string)  [unwired: 14 in]
      }
      frame "XY: Symmeterize" {
        # "Template Separator\n(You can make a copy of, or modify, this frame)"
        n250 = Unbundle By Name(w577) -> ("XY Data (processed 1)"=w578:cluster{"Intensity Data":dbl[], "Array":dbl[]}[])
        n251 = call-poly <userlib>:"Symmetrize.vi"("error in (no error)"=w574, "XY-data"=w578) -> ("error out"=w573:errorcluster, "Antisymmetric"=→"XY Graph: Antisymmetric":cluster{"X-array":dbl[], dbl[]}[], "Symmetric"=→"XY Graph: Symmetric":cluster{"X-array":dbl[], dbl[]}[], "XY-data out"=w575:cluster{"X-array":dbl[], "Y-array":dbl[]}[])  [unwired: 6 in]
        n252 = Bundle By Name(cluster=w577, "XY Data (processed 1)"=w575) -> (w576:T5)
        n253 = call <vilib>:"Add State(s) to Queue__JKI_lib_State_Machine.vi"("State(s) in (\"\")"=w580) -> ("States Out"=w579:string)  [unwired: 14 in]
      }
    }
  }
